vi "MultiPAS-UV-roll.vi"() -> ()   [LabVIEW 2011]
uses:
  sub/crd/fit/Analysis/analys_meth.ctl
  <vilib>/Analysis/4window.llb/windowTd.ctl
  sub/QMH/QMH Add Message to Queue (Single Element).vi
  sub/QMH/QMH Add Message to Queue (Array).vi
  sub/laserDiagnose_UV.vi
  <vilib>/Instr/_visa.llb/VISA Configure Serial Port (Instr).vi
  <vilib>/Utility/file.llb/Write To Spreadsheet File (string).vi
  sub/fftGetMags.vi
  sub/rollingAverage_III.vi
  sub/pdNormalize_III.vi
  <vilib>/measure/maspectr.llb/FFT Spectrum (Mag-Phase) for 1 Chan.vi
  sub/absCalcPlot_UV.vi
  sub/micUnbundle_III.vi
  <vilib>/measure/NI_MAPro.lvlib
  <vilib>/Analysis/NI_AALPro.lvlib
panel:
  out "x 2":dbl
  in  "x":dbl
  in  "y":dbl
  out "Chopper On":bool=TRUE caption="Overtemp"
  in  "Chopper":bool=TRUE
  in  "save spectrum":bool
  out "PAS Save":bool caption="Overtemp"
  in  "Data 2":i32[][](array[numeric])=[[-16374, -7248, 2543, 12030, 20279, 26487, 30037, 30583, 28073, 22744, 15131, 5976, -3818, -13288, -21504, -27663, -31155, -31636, -29064, -23686, -16036, -6862, 2936, 12388, 20571, 26684, 30122, 30546, 27911, 22483, 14793, 5595, -4207, -13644, -21795, -27855, -31232, -31591, -28898, -23423, -15695, -6476, 3323, 12743, 20858, 26873, 30194, 30492, 27744, 22213, 14447, 5207, -4597, -14002, -22082, -28044, -31304, -31540, -28731, -23149, -15348, -6093, 3713, 13101, 21145, 27063, 30265, 30442, 27576, 21943, 14103, 4822, -4984, -14354, -22365, -28230, -31373, -31485, -28556, -22876, -14998, -5702, 4104, 13452, 21428, 27245, 30335, 30388, 27400, 21669, 13754, 4435, -5375, -14705, -22643, -28407, -31436, -31426, -28378, -22598, -14648, -5314, 4497, 13803, 21706, 27423, 30394, 30325, 27221, 21390, 13402, 4045, -5763, -15056, -22921, -28586, -31496, -31361, -28198, -22319, -14297, -4924, 4879, 14151, 21982, 27597, 30451, 30257, 27038, 21107, 13050, 3658, -6149, -15402, -23193, -28754, -31546, -31290, -28010, -22033, -13944, -4536, 5266, 14498, 22252, 27767, 30500, 30184, 26849, 20821, 12696, 3267, -6535, -15748, -23462, -28924, -31596, -31216, -27821, -21748, -13587, -4147, 5653, 14838, 22519, 27930, 30549, 30110, 26658, 20535, 12337, 2878, -6919, -16089, -23727, -29087, -31641, -31137, -27627, -21457, -13229, -3753, 6038, 15181, 22786, 28093, 30591, 30031, 26461, 20243, 11979, 2485, -7303, -16428, -23991, -29244, -31678, -31053, -27426, -21159, -12867, -3360, 6424, 15524, 23043, 28252, 30633, 29946, 26262, 19946, 11617, 2096, -7686, -16764, -24246, -29398, -31712, -30964, -27224, -20862, -12503, -2971, 6803, 15859, 23301, 28401, 30661, 29852, 26058, 19648, 11254, 1703, -8069, -17099, -24500, -29547, -31741, -30870, -27018, -20562, -12138, -2575, 7188, 16192, 23556, 28549, 30689, 29756, 25848, 19348, 10891, 1312, -8448, -17430, -24753, -29691, -31765, -30773, -26806, -20259, -11775, -2186, 7566, 16521, 23801, 28690, 30709, 29656, 25634, 19038, 10523, 919, -8831, -17762, -24997, -29833, -31788, -30672, -26593, -19955, -11409, -1792, 7944, 16850, 24047, 28830, 30724, 29548, 25416, 18729, 10152, 523, -9212, -18092, -25245, -29969, -31805, -30566, -26375, -19647, -11041, -1403, 8319, 17173, 24287, 28963, 30734, 29436, 25192, 18418, 9781, 130, -9587, -18413, -25481, -30101, -31814, -30449, -26150, -19332, -10666, -1007, 8697, 17497, 24524, 29090, 30745, 29325, 24968, 18105, 9408, -263, -9962, -18735, -25718, -30228, -31820, -30334, -25921, -19016, -10296, -618, 9072, 17814, 24756, 29213, 30746, 29202, 24738, 17787, 9036, -657, -10338, -19058, -25951, -30350, -31818, -30214, -25690, -18699, -9922, -224, 9442, 18128, 24984, 29330, 30738, 29078, 24502, 17466, 8658, -1050, -10710, -19371, -26178, -30467, -31814, -30088, -25458, -18382, -9550, 167, 9812, 18440, 25206, 29443, 30732, 28947, 24264, 17143, 8281, -1445, -11083, -19685, -26404, -30581, -31807, -29959, -25221, -18059, -9175, 556, 10178, 18750, 25426, 29548, 30718, 28809, 24018, 16812, 7901, -1842, -11457, -19996, -26624, -30690, -31795, -29824, -24980, -17733, -8799, 950, 10549, 19058, 25643, 29655, 30700, 28673, 23773, 16484, 7523, -2235, -11824, -20304, -26840, -30793, -31772, -29682, -24731, -17402, -8415, 1341, 10916, 19363, 25856, 29755, 30677, 28528, 23522, 16151, 7141, -2626, -12191, -20607, -27051, -30891, -31746, -29536, -24481, -17070, -8035, 1733, 11280, 19664, 26064, 29851, 30648, 28381, 23272, 15818, 6762, -3019, -12555, -20906, -27258, -30984, -31717, -29391, -24226, -16736, -7655, 2128, 11641, 19962, 26270, 29940, 30615, 28229, 23013, 15483, 6376, -3409, -12914, -21204, -27459, -31071, -31684, -29236, -23967, -16398, -7271, 2515, 12005, 20258, 26468, 30024, 30577, 28072, 22753, 15143, 5990, -3802, -13276, -21497, -27660, -31157, -31643, -29076, -23707, -16058, -6886, 2908, 12363, 20550, 26666, 30107, 30536, 27914, 22489, 14805, 5607, -4192, -13633, -21787, -27849, -31230, -31597, -28911, -23438, -15716, -6501, 3298, 12719, 20839, 26858, 30182, 30488, 27744, 22223, 14459, 5225, -4579, -13988, -22071, -28040, -31304, -31549, -28743, -23167, -15368, -6113, 3693, 13076, 21126, 27047, 30255, 30438, 27576, 21950, 14113, 4837, -4971, -14340, -22354, -28224, -31375, -31494, -28570, -22895, -15022, -5725, 4080, 13430, 21408, 27230, 30324, 30384, 27402, 21676, 13766, 4449, -5360, -14694, -22636, -28409, -31440, -31436, -28397, -22617, -14674, -5338, 4467, 13781, 21686, 27408, 30385, 30320, 27224, 21398, 13418, 4062, -5748, -15044, -22913, -28584, -31498, -31368, -28212, -22339, -14321, -4948, 4856, 14131, 21963, 27583, 30440, 30254, 27042, 21118, 13062, 3669, -6137, -15390, -23183, -28751, -31551, -31297, -28024, -22049, -13962, -4556, 5245, 14476, 22235, 27754, 30497, 30186, 26857, 20834, 12710, 3283, -6519, -15733, -23453, -28921, -31600, -31226, -27837, -21765, -13610, -4168, 5628, 14820, 22502, 27918, 30540, 30109, 26664, 20544, 12354, 2891, -6906, -16074, -23719, -29085, -31646, -31148, -27642, -21475, -13251, -3777, 6014, 15160, 22765, 28078, 30583, 30027, 26468, 20251, 11994, 2501, -7292, -16415, -23980, -29242, -31682, -31064, -27443, -21181, -12892, -3386, 6397, 15501, 23026, 28238, 30624, 29944, 26269, 19959, 11633, 2110, -7673, -16753, -24239, -29395, -31719, -30974, -27239, -20882, -12528, -2993, 6782, 15835, 23285, 28390, 30651, 29852, 26063, 19660, 11271, 1720, -8053, -17087, -24493, -29546, -31746, -30880, -27031, -20583, -12163, -2599, 7166, 16173, 23538, 28538, 30684, 29758, 25853, 19356, 10906, 1327, -8433, -17416, -24743, -29688, -31769, -30782, -26821, -20280, -11797, -2208, 7543, 16501, 23786, 28680, 30704, 29656, 25642, 19053, 10540, 936, -8814, -17747, -24989, -29827, -31787, -30678, -26606, -19973, -11430, -1817, 7923, 16829, 24031, 28819, 30721, 29552, 25424, 18746, 10174, 543, -9191, -18072, -25231, -29962, -31802, -30567, -26384, -19660, -11057, -1422, 8302, 17159, 24274, 28952, 30738, 29443, 25205, 18435, 9801, 150, -9568, -18401, -25472, -30095, -31811, -30457, -26163, -19349, -10687, -1031, 8679, 17481, 24511, 29082, 30742, 29327, 24979, 18121, 9431, -241, -9943, -18717, -25707, -30221, -31815, -30337, -25930, -19029, -10312, -631, 9058, 17802, 24745, 29207, 30746, 29209, 24750, 17805, 9057, -634, -10316, -19037, -25937, -30340, -31814, -30217, -25700, -18713, -9939, -240, 9429, 18117, 24976, 29328, 30740, 29088, 24519, 17486, 8682, -1027, -10688, -19352, -26164, -30458, -31810, -30091, -25465, -18390, -9561, 154, 9800, 18433, 25201, 29442, 30735, 28959, 24282, 17165, 8308, -1420, -11063, -19665, -26386, -30570, -31801, -29961, -25227, -18068, -9185, 547, 10171, 18745, 25424, 29552, 30726, 28825, 24038, 16835, 7925, -1815, -11429, -19974, -26608, -30681, -31789, -29826, -24984, -17741, -8807, 938, 10536, 19047, 25636, 29657, 30708, 28685, 23794, 16510, 7550, -2205, -11798, -20280, -26821, -30782, -31766, -29684, -24737, -17411, -8429, 1331, 10906, 19356, 25851, 29758, 30684, 28544, 23546, 16178, 7169, -2598, -12162, -20582, -27035, -30879, -31744, -29540, -24485, -17080, -8048, 1721, 11267, 19655, 26061, 29852, 30654, 28395, 23291, 15843, 6786, -2993, -12527, -20884, -27240, -30974, -31713, -29390, -24230, -16744, -7662, 2115, 11635, 19957, 26268, 29945, 30624, 28246, 23035, 15509, 6406, -3382, -12889, -21180, -27444, -31061, -31677, -29236, -23975, -16408, -7284], [-19329, -1252, 17344, 29341, 30145, 19451, 1353, -17227, -29174, -29920, -19175, -1056, 17506, 29408, 30095, 19300, 1159, -17387, -29238, -29860, -19019, -860, 17671, 29475, 30037, 19143, 960, -17553, -29307, -29809, -18866, -664, 17832, 29545, 29987, 18991, 771, -17707, -29365, -29749, -18707, -466, 17992, 29605, 29926, 18832, 570, -17873, -29434, -29694, -18556, -272, 18151, 29670, 29869, 18676, 375, -18031, -29495, -29633, -18395, -75, 18310, 29729, 29809, 18516, 175, -18194, -29561, -29579, -18238, 120, 18469, 29792, 29750, 18362, -17, -18347, -29617, -29515, -18076, 316, 18629, 29848, 29682, 18197, -218, -18510, -29679, -29456, -17921, 513, 18787, 29910, 29626, 18042, -408, -18664, -29734, -29388, -17757, 709, 18941, 29965, 29560, 17875, -609, -18823, -29791, -29326, -17600, 904, 19095, 30023, 29495, 17717, -802, -18975, -29845, -29260, -17434, 1099, 19251, 30075, 29425, 17551, -1001, -19131, -29901, -29194, -17277, 1296, 19408, 30130, 29359, 17393, -1193, -19284, -29953, -29124, -17112, 1491, 19560, 30184, 29290, 17225, -1392, -19440, -30008, -29056, -16949, 1686, 19713, 30237, 29226, 17069, -1581, -19587, -30054, -28982, -16781, 1883, 19866, 30287, 29151, 16898, -1781, -19742, -30107, -28913, -16616, 2079, 20018, 30337, 29082, 16737, -1973, -19888, -30152, -28838, -16449, 2275, 20167, 30383, 29006, 16564, -2174, -20041, -30200, -28765, -16282, 2471, 20321, 30430, 28934, 16403, -2364, -20187, -30243, -28688, -16113, 2669, 20465, 30470, 28853, 16230, -2568, -20341, -30294, -28618, -15953, 2860, 20615, 30519, 28783, 16070, -2755, -20486, -30335, -28537, -15779, 3057, 20760, 30560, 28700, 15892, -2956, -20637, -30378, -28461, -15613, 3252, 20909, 30605, 28628, 15730, -3145, -20777, -30418, -28377, -15440, 3446, 21054, 30645, 28543, 15557, -3345, -20927, -30460, -28299, -15271, 3643, 21199, 30686, 28465, 15391, -3534, -21066, -30495, -28215, -15100, 3839, 21345, 30722, 28380, 15214, -3734, -21213, -30534, -28134, -14928, 4032, 21487, 30760, 28300, 15044, -3926, -21355, -30570, -28052, -14757, 4225, 21627, 30792, 28209, 14870, -4123, -21501, -30607, -27968, -14586, 4419, 21768, 30832, 28129, 14702, -4314, -21637, -30639, -27880, -14413, 4612, 21907, 30859, 28040, 14521, -4515, -21780, -30675, -27796, -14241, 4804, 22048, 30895, 27953, 14352, -4702, -21919, -30705, -27707, -14064, 4999, 22187, 30922, 27859, 14172, -4900, -22060, -30739, -27620, -13892, 5193, 22326, 30954, 27773, 14003, -5090, -22194, -30765, -27524, -13712, 5386, 22462, 30981, 27679, 13823, -5285, -22333, -30794, -27436, -13538, 5580, 22600, 31013, 27591, 13650, -5476, -22466, -30820, -27343, -13363, 5770, 22732, 31033, 27491, 13468, -5673, -22605, -30848, -27251, -13187, 5964, 22870, 31060, 27401, 13292, -5863, -22736, -30870, -27155, -13010, 6156, 23000, 31079, 27299, 13111, -6058, -22873, -30895, -27060, -12833, 6347, 23134, 31104, 27208, 12936, -6248, -23004, -30918, -26965, -12652, 6536, 23260, 31120, 27106, 12753, -6444, -23136, -30939, -26865, -12472, 6729, 23395, 31148, 27011, 12578, -6634, -23266, -30959, -26766, -12296, 6919, 23523, 31161, 26907, 12392, -6830, -23402, -30982, -26665, -12115, 7109, 23652, 31180, 26809, 12213, -7016, -23524, -30992, -26564, -11932, 7301, 23777, 31195, 26704, 12032, -7210, -23655, -31011, -26464, -11755, 7492, 23907, 31211, 26605, 11855, -7395, -23778, -31024, -26358, -11573, 7680, 24031, 31218, 26494, 11665, -7592, -23908, -31039, -26258, -11392, 7871, 24158, 31237, 26394, 11491, -7775, -24031, -31050, -26153, -11210, 8063, 24281, 31247, 26285, 11302, -7972, -24159, -31062, -26046, -11027, 8250, 24407, 31258, 26180, 11124, -8157, -24276, -31067, -25937, -10841, 8438, 24526, 31265, 26071, 10936, -8347, -24401, -31078, -25829, -10659, 8630, 24649, 31275, 25965, 10755, -8533, -24522, -31087, -25721, -10474, 8816, 24770, 31280, 25853, 10566, -8726, -24641, -31091, -25608, -10290, 9003, 24891, 31287, 25746, 10386, -8910, -24756, -31095, -25498, -10105, 9192, 25008, 31287, 25627, 10196, -9102, -24881, -31101, -25386, -9919, 9381, 25127, 31296, 25521, 10019, -9284, -24994, -31099, -25268, -9732, 9570, 25243, 31293, 25403, 9826, -9476, -25113, -31105, -25157, -9544, 9756, 25359, 31298, 25291, 9645, -9655, -25225, -31099, -25040, -9359, 9942, 25473, 31291, 25167, 9453, -9847, -25341, -31102, -24926, -9173, 10124, 25586, 31294, 25057, 9269, -10029, -25450, -31095, -24809, -8986, 10310, 25696, 31284, 24931, 9078, -10218, -25564, -31094, -24688, -8798, 10497, 25812, 31287, 24819, 8896, -10399, -25673, -31085, -24567, -8608, 10682, 25922, 31278, 24698, 8703, -10587, -25785, -31080, -24448, -8422, 10866, 26033, 31274, 24582, 8522, -10765, -25890, -31067, -24321, -8230, 11050, 26140, 31263, 24455, 8325, -10952, -26001, -31064, -24201, -8040, 11234, 26248, 31255, 24338, 8142, -11132, -26106, -31054, -24079, -7852, 11417, 26353, 31243, 24207, 7948, -11316, -26217, -31041, -23952, -7662, 11601, 26464, 31236, 24089, 7763, -11494, -26315, -31025, -23829, -7471, 11782, 26562, 31217, 23957, 7567, -11682, -26422, -31014, -23702, -7282, 11962, 26667, 31205, 23834, 7383, -11859, -26521, -30998, -23575, -7092, 12144, 26770, 31187, 23704, 7186, -12043, -26626, -30981, -23444, -6900, 12328, 26875, 31176, 23582, 7003, -12218, -26724, -30962, -23316, -6709, 12505, 26971, 31154, 23446, 6805, -12401, -26825, -30946, -23189, -6517, 12687, 27073, 31139, 23322, 6620, -12576, -26919, -30922, -23054, -6323, 12867, 27170, 31114, 23185, 6422, -12760, -27022, -30904, -22923, -6132, 13047, 27272, 31096, 23060, 6237, -12934, -27114, -30879, -22790, -5940, 13222, 27362, 31068, 22921, 6041, -13116, -27212, -30855, -22657, -5748, 13401, 27461, 31048, 22790, 5853, -13289, -27302, -30828, -22522, -5555, 13577, 27549, 31019, 22652, 5652, -13472, -27398, -30806, -22388, -5362, 13753, 27645, 30995, 22521, 5463, -13642, -27487, -30776, -22248, -5169, 13928, 27733, 30963, 22376, 5266, -13823, -27584, -30750, -22113, -4975, 14106, 27828, 30937, 22246, 5082, -13992, -27669, -30717, -21974, -4782, 14280, 27914, 30902, 22101, 4880, -14174, -27760, -30689, -21837, -4588, 14454, 28006, 30875, 21965, 4692, -14340, -27843, -30653, -21693, -4391, 14631, 28092, 30840, 21822, 4494, -14519, -27934, -30620, -21552, -4198, 14805, 28179, 30808, 21688, 4308, -14687, -28015, -30582, -21410, -4004, 14975, 28262, 30770, 21540, 4106, -14861, -28103, -30548, -21268, -3808, 15149, 28349, 30739, 21402, 3916, -15032, -28183, -30512, -21124, -3614, 15319, 28430, 30697, 21255, 3715, -15205, -28267, -30475, -20982, -3421, 15490, 28513, 30664, 21116, 3524, -15376, -28348, -30435, -20837, -3225, 15660, 28592, 30617, 20962, 3327, -15550, -28432, -30397, -20695, -3032, 15829, 28673, 30581, 20820, 3134, -15711, -28506, -30353, -20546, -2837, 15994, 28746, 30530, 20669, 2933, -15887, -28585, -30311, -20400, -2641, 16167, 28828, 30496, 20528, 2745, -16052, -28660, -30264, -20248, -2445, 16335, 28901, 30445, 20376, 2544, -16221, -28737, -30219, -20102, -2250, 16505, 28983, 30406, 20231, 2357, -16381, -28808, -30171, -19950, -2053, 16670, 29053, 30355, 20075, 2154, -16552, -28883, -30127, -19803, -1859, 16835, 29128, 30308, 19930, 1965, -16714, -28952, -30073, -19650, -1663, 17001, 29192, 30255, 19772, 1764, -16881, -29028, -30026, -19496, -1467, 17165, 29268, 30208, 19626, 1572, -17043, -29095, -29977, -19346]]
  out "Filtering":bool caption="Time has Elapsed"
  in  "Switch Filter":bool
  in  "Auto Filter":bool
  out "Elapsed Time (min)":dbl caption="Elapsed Time (s)" format="%#.1g"
  in  "Filter Length (min)":dbl=6.0 caption="Time Target (s)"
  in  "Sample Length (min)":dbl=24.0 caption="Time Target (s)" format="%#.1f"
  out "Time has Elapsed":bool
  in  "Time Target (s)":dbl=1.0
  in  "All Emit":bool
  in  "Alignment Mode":bool
  in  "445 Emission":bool
  in  "445 Power (mW)":dbl(slide)=75.0 min=0.0 max=75.0 step=1.0 scale=0.0..75.0
  in  "375 Emission":bool
  in  "375 Power (mW)":dbl(slide)=100.0 min=0.0 max=50.0 step=1.0 scale=0.0..50.0
  in  "320 Emission":bool=TRUE
  out "Overtemp":bool
  in  "Tab Control":T1(tab)=enum."Oscilloscope"
  out "Laser Currents":T2(graph)
  in  "Chopper Port":refnum<visa-resource-name>="COM6"
  out "sweeps":path caption="Microphone File Path"
  in  "save interval (ms)":u32=1000
  out "Error Console":T3
  out "pas":path caption="Microphone File Path"
  out "Laser Temperatures":T2(graph)
  in  "pd id":u32=2
  in  "mic id":u32
  in  "mic cal, scu":dbl=5.41531278804282e-05 format="%#_3e"
  in  "mic cal, scu":dbl=5.59307241877627e-05 format="%#_3e"
  in  "320 Port":refnum<visa-resource-name>="COM5"
  in  "375 Port":refnum<visa-resource-name>="COM14"
  in  "445 Port":refnum<visa-resource-name>="COM13"
  in  "Teensy Port":refnum<visa-resource-name>="COM12"
  in  "Save Data":bool
  in  "405 PD Cal 3":dbl=0.039
  in  "532 PD Cal 3":dbl=0.0348
  in  "660 PD Cal 3":dbl=0.2015
  out "Laser Powers":T2(graph)
  in  "tau Rolling Avg":i32=8
  out "error out":errorcluster
  in  "Channel B Settings":T4={"Enabled"=TRUE, "Coupling"=1, "Range"=8, "Analogue Offset"=0.0} {"Range" items=["20 mV"=1, "50 mV"=2, "100 mV"=3, "200 mV"=4, "500 mV"=5, "1 V"=6, "2 V"=7, "5 V"=8, "10 V"=9, "20 V"=10]; "Coupling" items=["AC", "DC"]}
  in  "Rapid Block Acquisition Settings":T5={"preTriggerSamples"=0, "postTriggerSamples"=90000, "timebase"=1, "Down-Sample Mode"=4, "Down Sample Ratio"=10, "Oversample"=1, "Number of Captures"=100} {"Down Sample Ratio" min=1 step=1; "Down-Sample Mode" items=["None"=0, "Aggregate"=1, "Decimate"=2, "Average"=4]}
  in  "crd delay":u32=1000
  in  "Trigger Settings":T6={"Trigger Enabled"=TRUE, "Trigger Source"=enum."Channel B", "Trigger Threshold (Volts)"=1.0, "Trigger Direction"=3, "Trigger Delay (samples)"=0, "Auto Trigger Time (ms)"=1000} {"Trigger Direction" items=["Rising"=2, "Falling"=3]}
  in  "Channel A Settings":T4={"Enabled"=TRUE, "Coupling"=0, "Range"=3, "Analogue Offset"=0.0} {"Range" items=["20 mV"=1, "50 mV"=2, "100 mV"=3, "200 mV"=4, "500 mV"=5, "1 V"=6, "2 V"=7, "5 V"=8, "10 V"=9, "20 V"=10]; "Coupling" items=["AC", "DC"]}
  in  "factor":sgl=10.0
  in  "sweep":bool
  out "freqscan":cluster{i32[], "Best Gaussian Fit":dbl[]}[](graph) caption="Frequency Sweep"
  out "sweep progress":dbl(slide) scale=0.0..1.0
  in  "Autosweep?":bool=TRUE
  in  "set freqs":bool
  out "Calculated Resonance (Hz)":dbl=1370.0
  in  "Data Start Frequency (Hz)":i32=1355
  in  "Data End Frequency (Hz)":i32=1405
  in  "320 F (Hz)":i32=1368
  in  "375 F (Hz)":i32=1372
  in  "445 F (Hz)":i32=1370
  in  "Chart Rolling Average":i32=16
  out "pdwave":waveform(i32)(graph) caption="Photodiode Waveform"
  out "pd ts":cluster{dbl, dbl, dbl}(graph)
  out "pdfft":cluster{"f0":dbl, "df":dbl, "magnitude":dbl[]}(graph) caption="Photodiode FFT"
  in  "rollavg":i32=16 caption="Dispaly Averaging (Transfers to Absorption Data!)"
  out "mic ts":T7(graph)
  out "micfft":cluster{"f0":dbl, "df":dbl, "magnitude":dbl[]}(graph) caption="Photodiode FFT"
  out "micwave":waveform(i32)(graph) caption="Photodiode Waveform"
  in  "tau0":dbl
  in  "getbkg":bool
  out "AAE":dbl(graph)
  in  "Bkg Values (mV)":cluster{dbl, dbl, dbl}
  out "Absorption Spectrum":cluster{dbl[], "Best Power Fit":dbl[]}[](graph)
  in  "cellcal":dbl=95000.0 caption="Cell Calibration Coefficient (mV/mW)"
  out "abs/ext":cluster{dbl, dbl, dbl, "b_ext (1/Mm)":dbl}(graph)
  out "tau":dbl(graph)
  out "decay":cluster{i32, dbl, "Data (mV)":dbl[]}[](graph)
  out "Status":string
  in  "Exit":bool
  in  "State Variables":cluster{"CurrentFile":path}
  # "MultiPAS-UV | AeroSmith Labs (2017)"
  # "Laser Control"
  # "Filter Control"
  # "Communications"
  # "Sound Card Parameters"
  # "Data File Options"
  # "File paths are populated automatically at <...\\My Documents\\MultiPAS Data\\>.  To save in another location, turn on \"Save Data\" and follow the prompts to choose an alternate working directory."
  # "Photodiode Calibration"
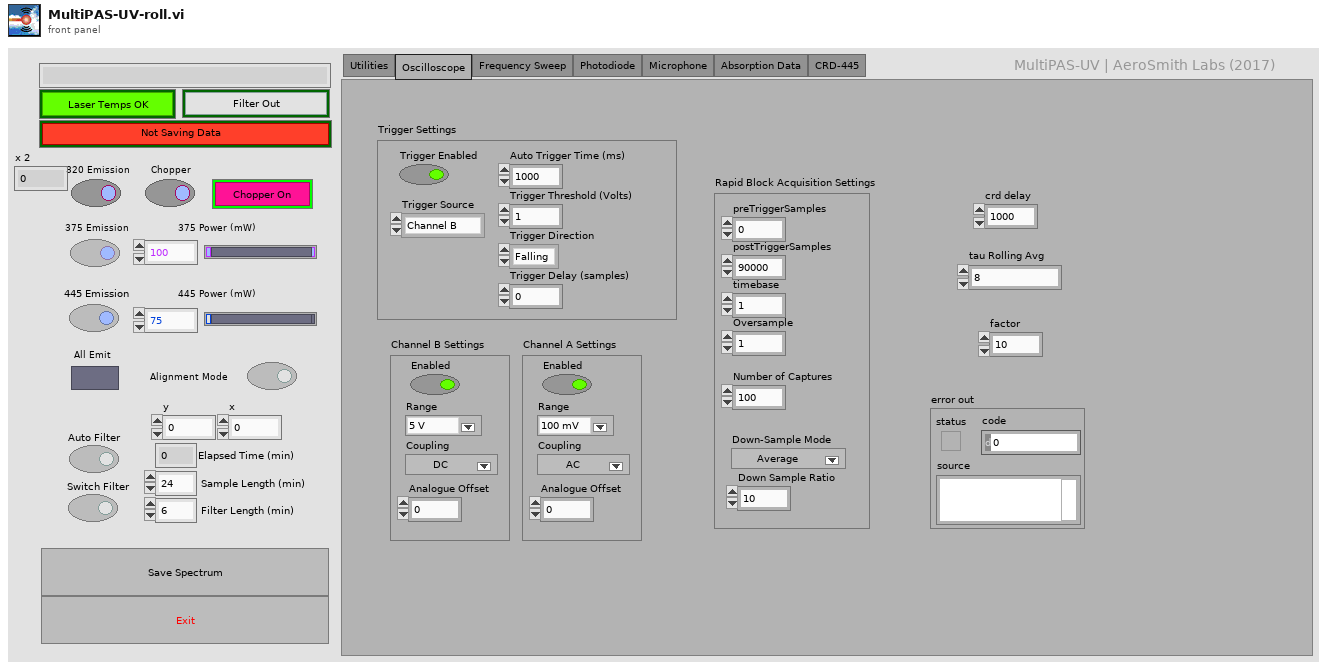
[diagram p1: front panel]
types:
  T1 = enum32{"Utilities", "Oscilloscope", "Frequency Sweep", "Photodiode", "Microphone", "Absorption Data", "CRD-445"}
  T2 = cluster{"Temp (C)":dbl, "Temp (C)":dbl, "Temp (C)":dbl}
  T3 = cluster{"status":bool, "code":i32, "Message":string}
  T4 = cluster{"Enabled":bool, "Coupling":i16, "Range":u16, "Analogue Offset":sgl}
  T5 = cluster{"preTriggerSamples":u32, "postTriggerSamples":u32, "timebase":u32, "Down-Sample Mode":i32, "Down Sample Ratio":u32, "Oversample":i16, "Number of Captures":u32}
  T6 = cluster{"Trigger Enabled":bool, "Trigger Source":enum16{"Channel A", "Channel B", "Channel C", "Channel D", "Ext."}, "Trigger Threshold (Volts)":dbl, "Trigger Direction":u16, "Trigger Delay (samples)":u32, "Auto Trigger Time (ms)":i16}
  T7 = cluster{"422 Mean":dbl, "532 Mean":dbl, "785 Mean":dbl}
  T8 = cluster{"# buffers":i32, "Buffer size":i32, "unit (ms)":enum16{"time (ms)", "Samples"}}
  T9 = typedef "SoundHandle.ctl" = cluster{"DeviceID":u16, "Samples/buf":u32, "Sampl rate":u32, "Bits/sample":u16, "Channels":u8, "Opened":bool}
  T10 = cluster{"Output Power at Laser Head":dbl, "Output Power at Laser Head":dbl, "Output Power at Laser Head":dbl}
  T11 = cluster{"Current (mA)":dbl, "Current (mA)":dbl, "Current (mA)":dbl}
  T12 = cluster{"405 Mean":dbl, "532 Mean":dbl, "660 Mean":dbl}
  T13 = typedef "NI_AALPro.lvlib/windowTd.ctl" = u32
  T14 = cluster{"785 New Array":dbl[], "785 Mean":dbl, "785 SD":dbl}
  T15 = cluster{"532 New Array":dbl[], "532 Mean":dbl, "532 SD":dbl}
  T16 = cluster{"422 New Array":dbl[], "422 Mean":dbl, "422 SD":dbl}
  T17 = typedef "analys_meth.ctl" = enum16{"DFT-1", "DFT-5", "LRS"}
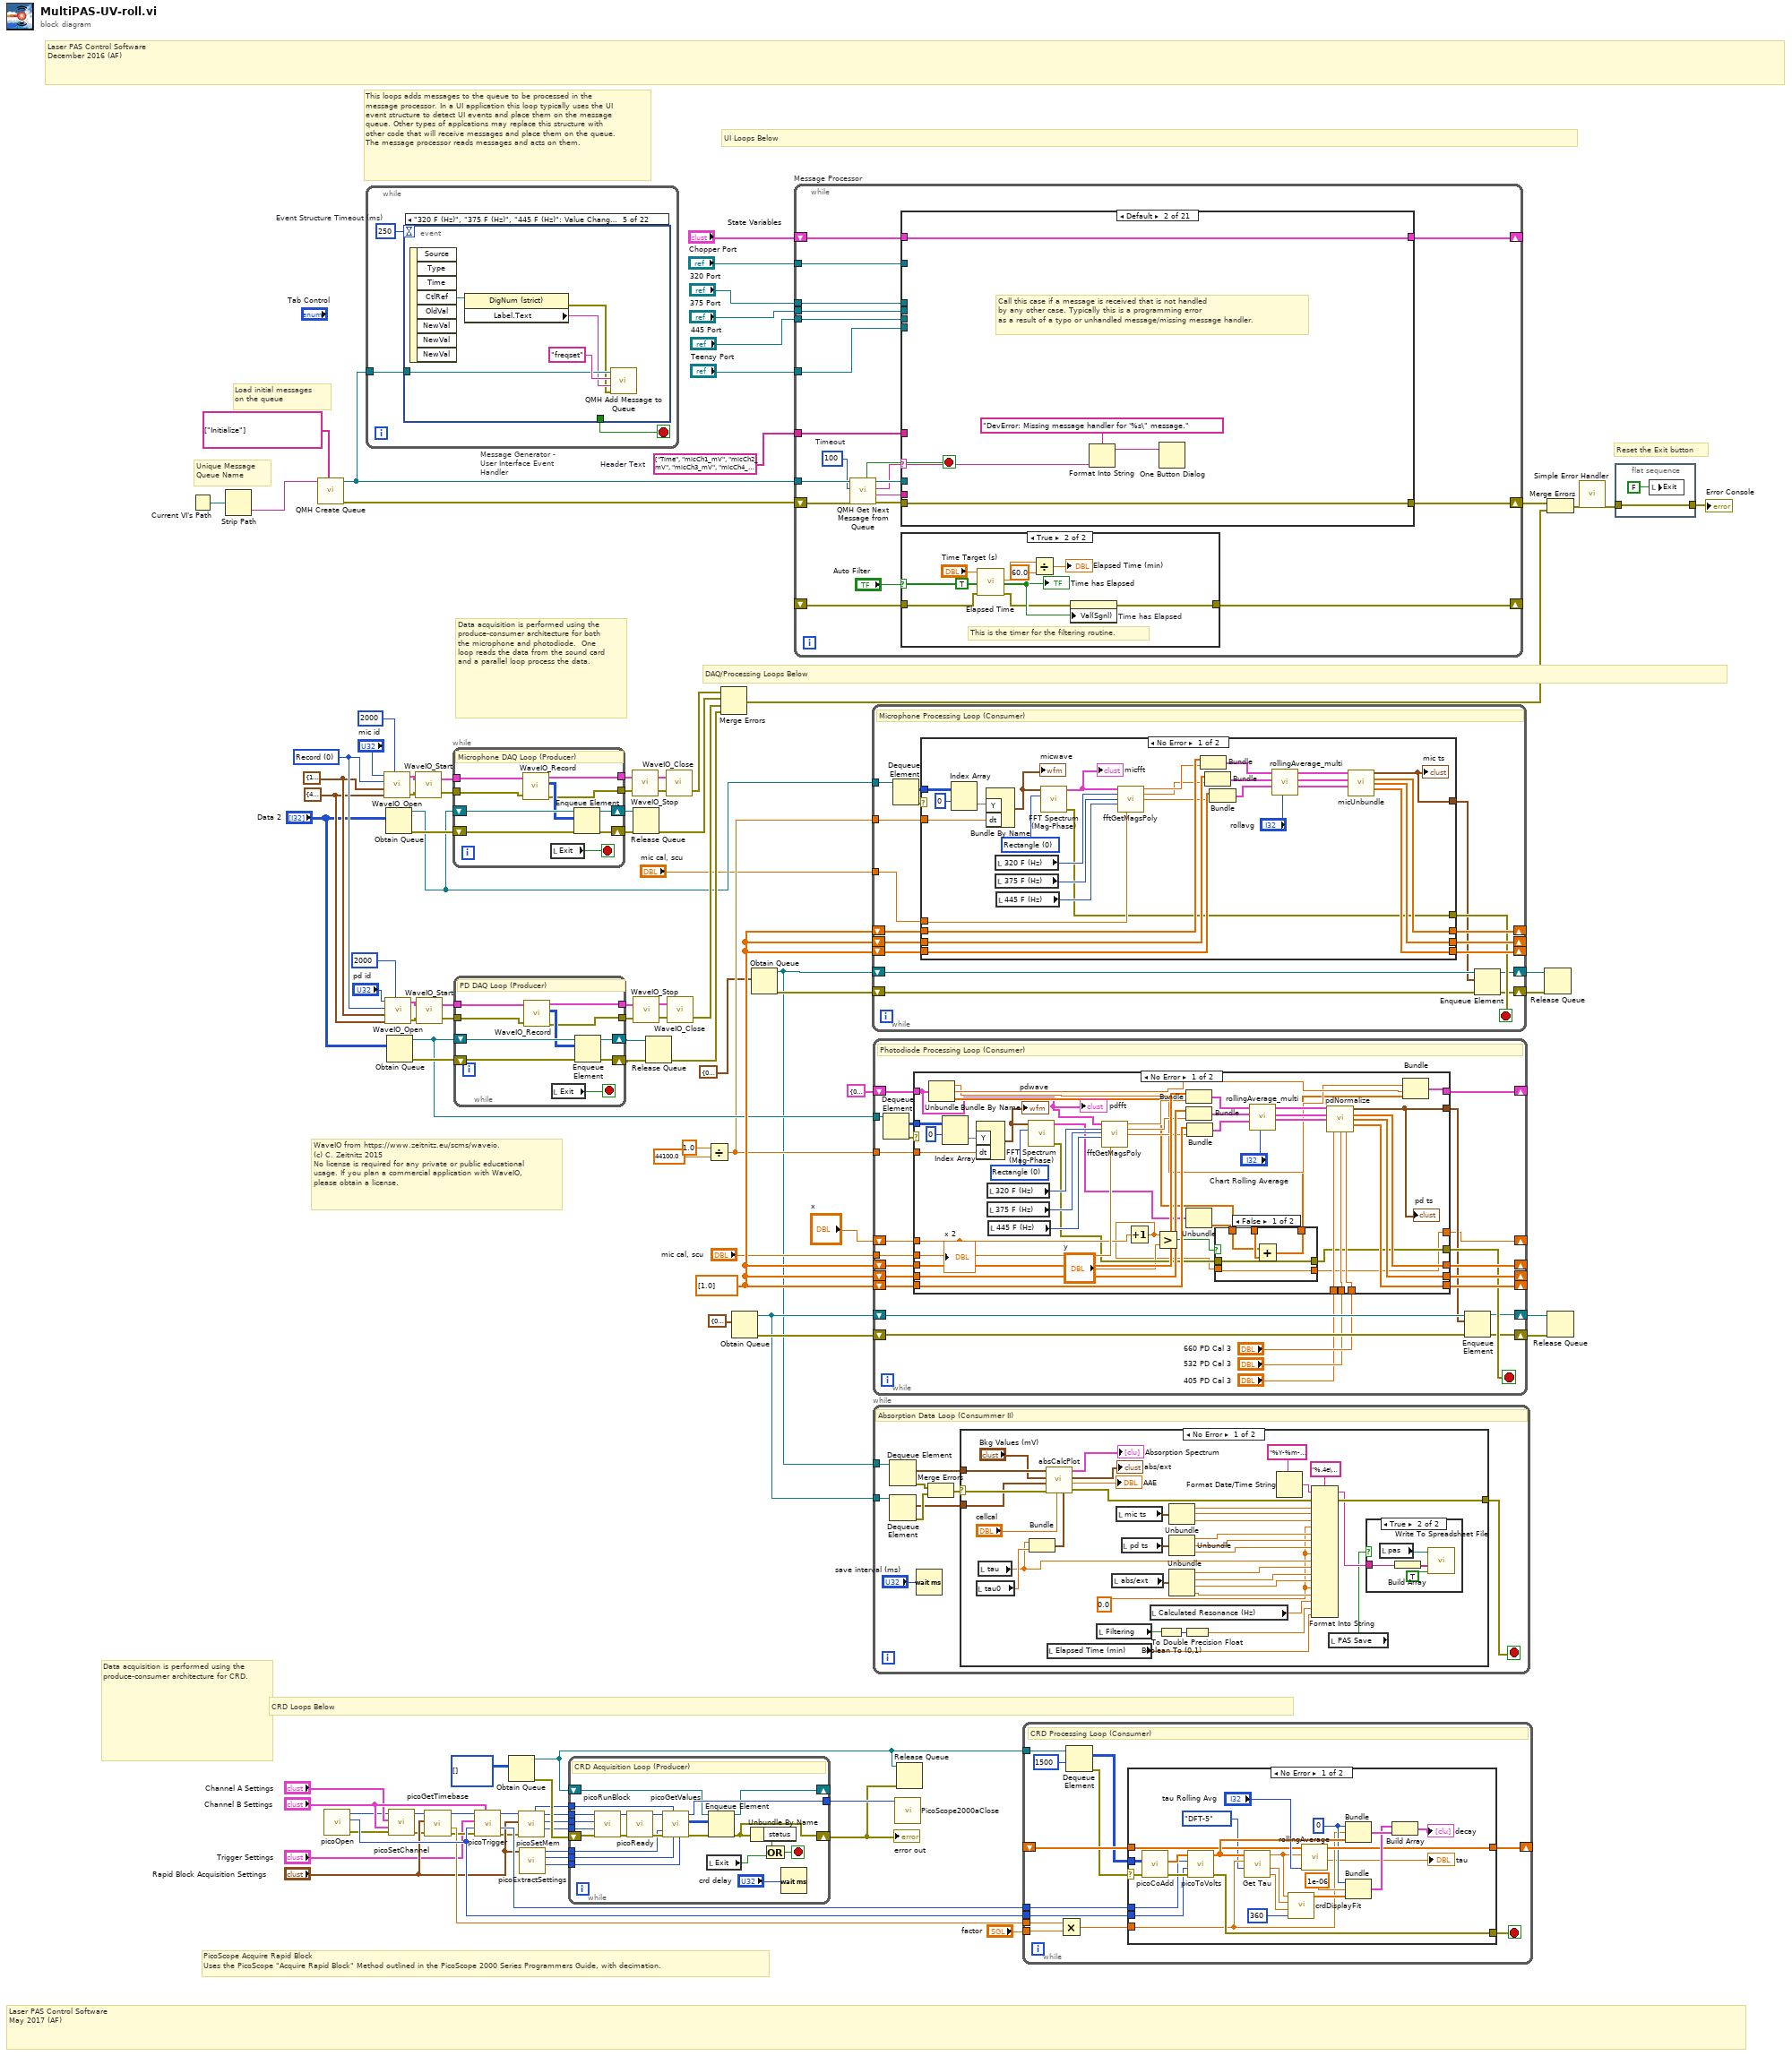
[diagram p0: block diagram]
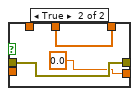
[diagram p5: hidden frame]
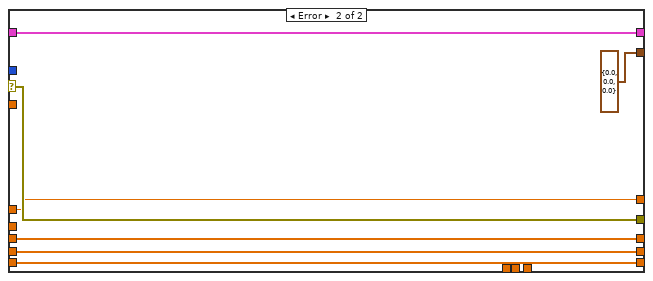
[diagram p6: hidden frame]
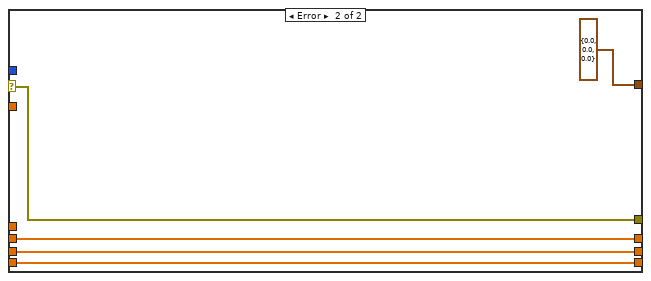
[diagram p7: hidden frame]
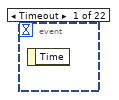
[diagram p8: hidden frame]
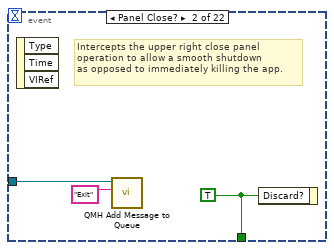
[diagram p9: hidden frame]
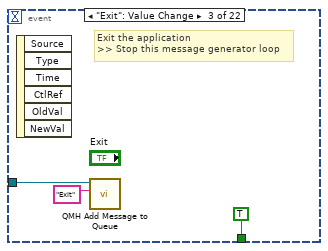
[diagram p10: hidden frame]
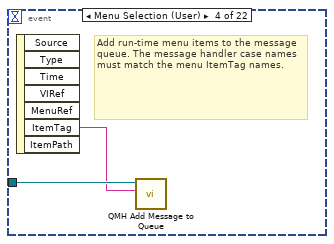
[diagram p11: hidden frame]
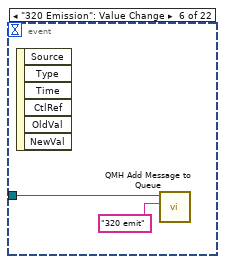
[diagram p12: hidden frame]
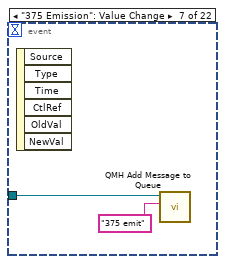
[diagram p13: hidden frame]
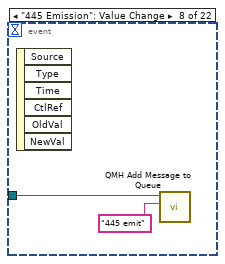
[diagram p14: hidden frame]
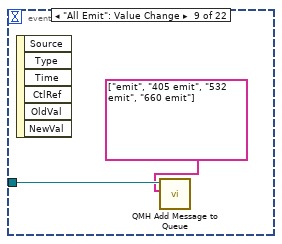
[diagram p15: hidden frame]
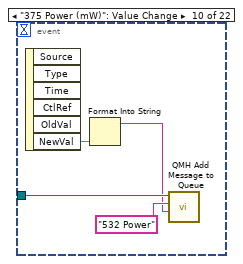
[diagram p16: hidden frame]
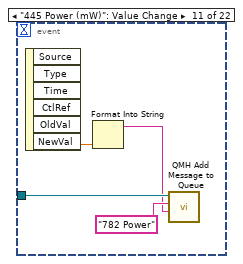
[diagram p17: hidden frame]
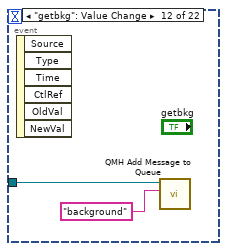
[diagram p18: hidden frame]
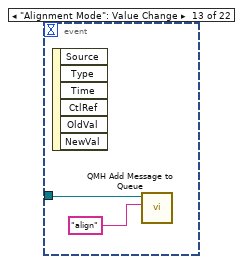
[diagram p19: hidden frame]
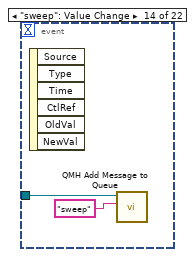
[diagram p20: hidden frame]
diagram:
  w32 = string[] ["Time", "micCh1_mV", "micCh2_mV", "micCh3_mV", "micCh4_mV", "pdCh1_mV", "pdCh2_mV", "pdCh3_mV", "pdCh4_mV", "tau_sec", "babsCh1_Mm", "babsCh2_Mm", "babsCh3_Mm", "babsCh4_Mm", "bext_Mm", "fres_Hz", "filter_state", "elapsedTime_min"]  # Header Text
  w52 = T8 {"# buffers"=10, "Buffer size"=44100, "unit (ms)"=enum."Samples"} ("Buffer")
  w51 = cluster{"Rate":i32, "Bits":i32, "Channels":i32} {"Rate"=44100, "Bits"=24, "Channels"=2} ("Format")
  w53 = u16 0 items=["Record", "Play", "Loopback", "ASIO input", "ASIO output"] ("Direction (Record)")
  w83 = dbl[] [1.0] ("X")
  # "PicoScope Acquire Rapid Block\nUses the PicoScope \"Acquire Rapid Block\" Method outlined in the PicoScope 2000 Series Programmers Guide, with decimation."
  # "Data acquisition is performed using the produce-consumer architecture for CRD."
  # "CRD Loops Below"
  # "Laser PAS Control Software\nMay 2017 (AF)"
  # "Laser PAS Control Software\nDecember 2016 (AF)"
  # "Data acquisition is performed using the produce-consumer architecture for both the microphone and photodiode.  One loop reads the data from the sound card and a parallel loop process the data."
  # "WaveIO from https://www.zeitnitz.eu/scms/waveio.\n(c) C. Zeitnitz 2015\nNo license is required for any private or public educational usage. If you plan a commercial application with WaveIO, please obtain a license."
  # "This loops adds messages to the queue to be processed in the message processor. In a UI application this loop typically uses the UI event structure to detect UI events and place them on the message queue. Other types of applcations may replace this structure with other code that will receive messages and place them on the queue.  The message processor reads messages and acts on them."
  # "Reset the Exit button"
  # "Unique Message\nQueue Name"
  # "Load initial messages\non the queue"
  # "DAQ/Processing Loops Below"
  # "UI Loops Below"
  n1 = Current VI's Path() -> (path=w98:path)
  n2 = Strip Path(path=w98) -> (name=w99:string)  [unwired: 1 out]
  n3 = call "QMH Create Queue.vi"("Initial Messages"=string[] ["Initialize"], "Message queue name (unnamed)"=w99) -> ("error out"=w95:errorcluster, "queue out"=w80:refnum<queue>)  [unwired: 8 in]
  n4 = call "picoOpen.vi"() -> ("error out"=w7:errorcluster, "maxADC"=w26:i16, "Handle Out"=w6:i16)  [unwired: 8 in, 1 out]
  n5 = while "Message Generator - User Interface Event Handler" {
    tunnel: w80 -> [w100]
    stop <- w101 stop-if-true
    w102 = 250  # Event Structure Timeout (ms)
    n6 = event shown="[4] \"320 F (Hz)\", \"375 F (Hz)\", \"445 F (Hz)\": Value Change" {
      selector: _ -> [_ _ _ _ _ _ _ _ _ _ _ _ _ _ _ _ _ _ _ _ _ _]
      dyn-events: _ -> [_ _ _ _ _ _ _ _ _ _ _ _ _ _ _ _ _ _ _ _ _ _]
      timeout: w102 -> [_ _ _ _ _ _ _ _ _ _ _ _ _ _ _ _ _ _ _ _ _ _]
      tunnel: [_ w105 TRUE ("Discard?") _ _ _ _ _ _ _ _ _ _ _ _ _ _ _ _ _ _ _] -> w101
      tunnel: w100 -> [_ w104 w107 w110 w114 w116 w118 w120 w123 w126 w130 w132 w134 w137 w141 w146 w151 w155 w160 w162 w164 w166]
      event Timeout {
        n7 = event-data() -> ()  [unwired: 1 in, 1 out]
      }
      event Panel Close? {
        w105 = TRUE ("Discard?")
        # "Intercepts the upper right close panel\noperation to allow a smooth shutdown\nas opposed to immediately killing the app."
        n8 = event-data() -> ()  [unwired: 1 in, 3 out]
        n9 = call-poly "QMH Add Message to Queue.vi"("Message"="Exit", "queue in"=w104) -> ()  [unwired: 8 in, 2 out]
        n10 = event-data("Discard?"=w105) -> ()  [unwired: 1 in, 1 out]
      }
      event "Exit": Value Change {
        # "Exit the application\n>> Stop this message generator loop"
        n11 = event-data() -> ()  [unwired: 1 in, 6 out]
        n12 = call-poly "QMH Add Message to Queue.vi"("Message"="Exit", "queue in"=w107) -> ()  [unwired: 8 in, 2 out]
      }
      event Menu Selection (User) {
        # "Add run-time menu items to the message\nqueue. The message handler case names must match the menu ItemTag names."
        n13 = event-data() -> ("ItemTag"=w109:string)  [unwired: 1 in, 6 out]
        n14 = call-poly "QMH Add Message to Queue.vi"("Message"=w109, "queue in"=w110) -> ()  [unwired: 8 in, 2 out]
      }
      event "320 F (Hz)", "375 F (Hz)", "445 F (Hz)": Value Change {
        n15 = event-data() -> ("CtlRef"=w113:refnum<vi>)  [unwired: 1 in, 7 out]
        n16 = property class="DigNum (strict)"(reference=w113) -> (error out=w111:errorcluster, "Label.Text"=w112:string)  [unwired: 1 in, 1 out]
        n17 = call-poly "QMH Add Message to Queue.vi"("error in (no error)"=w111, "Parameter"=w112, "Message"="freqset", "queue in"=w114) -> ()  [unwired: 6 in, 2 out]
      }
      event "320 Emission": Value Change {
        n18 = event-data() -> ()  [unwired: 1 in, 6 out]
        n19 = call-poly "QMH Add Message to Queue.vi"("Message"="320 emit", "queue in"=w116) -> ()  [unwired: 8 in, 2 out]
      }
      event "375 Emission": Value Change {
        n20 = event-data() -> ()  [unwired: 1 in, 6 out]
        n21 = call-poly "QMH Add Message to Queue.vi"("Message"="375 emit", "queue in"=w118) -> ()  [unwired: 8 in, 2 out]
      }
      event "445 Emission": Value Change {
        n22 = event-data() -> ()  [unwired: 1 in, 6 out]
        n23 = call-poly "QMH Add Message to Queue.vi"("Message"="445 emit", "queue in"=w120) -> ()  [unwired: 8 in, 2 out]
      }
      event "All Emit": Value Change {
        n24 = event-data() -> ()  [unwired: 1 in, 6 out]
        n25 = call-poly "QMH Add Message to Queue.vi"("Messages"=string[] ["emit", "405 emit", "532 emit", "660 emit"], "queue in"=w123) -> ()  [unwired: 8 in, 2 out]
      }
      event "375 Power (mW)": Value Change {
        n26 = event-data() -> ("NewVal"=w125:dbl)  [unwired: 1 in, 5 out]
        n27 = Format Into String(w125) -> (resulting string=w124:string)  [unwired: 3 in, 1 out]
        n28 = call-poly "QMH Add Message to Queue.vi"("Parameter"=w124, "Message"="532 Power", "queue in"=w126) -> ()  [unwired: 7 in, 2 out]
      }
      event "445 Power (mW)": Value Change {
        n29 = event-data() -> ("NewVal"=w129:dbl)  [unwired: 1 in, 5 out]
        n30 = Format Into String(w129) -> (resulting string=w128:string)  [unwired: 3 in, 1 out]
        n31 = call-poly "QMH Add Message to Queue.vi"("Parameter"=w128, "Message"="782 Power", "queue in"=w130) -> ()  [unwired: 7 in, 2 out]
      }
      event "getbkg": Value Change {
        n32 = event-data() -> ()  [unwired: 1 in, 6 out]
        n33 = call-poly "QMH Add Message to Queue.vi"("Message"="background", "queue in"=w132) -> ()  [unwired: 8 in, 2 out]
      }
      event "Alignment Mode": Value Change {
        n34 = event-data() -> ()  [unwired: 1 in, 6 out]
        n35 = call-poly "QMH Add Message to Queue.vi"("Message"="align", "queue in"=w134) -> ()  [unwired: 8 in, 2 out]
      }
      event "sweep": Value Change {
        n36 = event-data() -> ()  [unwired: 1 in, 6 out]
        n37 = call-poly "QMH Add Message to Queue.vi"("Message"="sweep", "queue in"=w137) -> ()  [unwired: 8 in, 2 out]
      }
      event "set freqs": Value Change {
        n38 = event-data() -> ()  [unwired: 1 in, 6 out]
        n39 = local read "Calculated Resonance (Hz)"() -> (w140:dbl)
        n40 = Format Into String(w140) -> (resulting string=w139:string, error out=w138:errorcluster)  [unwired: 3 in]
        n41 = call-poly "QMH Add Message to Queue.vi"("error in (no error)"=w138, "Parameter"=w139, "Message"="setfreqs", "queue in"=w141) -> ()  [unwired: 6 in, 2 out]
      }
      event "Save Data": Value Change {
        n42 = event-data() -> ("NewVal"=w145:bool)  [unwired: 1 in, 5 out]
        n43 = Format Into String(w145) -> (resulting string=w144:string, error out=w143:errorcluster)  [unwired: 3 in]
        n44 = call-poly "QMH Add Message to Queue.vi"("error in (no error)"=w143, "Parameter"=w144, "Message"="namefiles", "queue in"=w146) -> ()  [unwired: 6 in, 2 out]
      }
      event "Switch Filter": Value Change {
        n45 = event-data() -> ("NewVal"=w150:bool)  [unwired: 1 in, 5 out]
        n46 = local write "Filtering"(w150) -> ()
        n47 = Format Into String(w150) -> (resulting string=w148:string)  [unwired: 3 in, 1 out]
        n48 = call-poly "QMH Add Message to Queue.vi"("Parameter"=w148, "Message"="filterswitch", "queue in"=w151) -> ()  [unwired: 7 in, 2 out]
      }
      event "Time has Elapsed": Value Change {
        n49 = event-data() -> ("NewVal"=w154:bool)  [unwired: 1 in, 5 out]
        n50 = local read "Filtering"() -> (w153:bool)
        n51 = call "filterCreateMsg.vi"("time elapsed?"=w154, "auto sweep (true)"="Autosweep?", "filtering (true)"=w153, "queue in"=w155) -> ()  [unwired: 6 in, 2 out]
      }
      event "Calculated Resonance (Hz)": Value Change {
        n52 = event-data() -> ("NewVal"=w158:dbl)  [unwired: 1 in, 5 out]
        n53 = Format Into String(w158) -> (resulting string=w156:string, error out=w157:errorcluster)  [unwired: 3 in]
        n54 = call-poly "QMH Add Message to Queue.vi"("error in (no error)"=w157, "Parameter"=w156, "Message"="setfreqs", "queue in"=w160) -> ()  [unwired: 6 in, 2 out]
      }
      event "PAS Save": Value Change {
        n55 = event-data() -> ()  [unwired: 1 in, 6 out]
        n56 = call-poly "QMH Add Message to Queue.vi"("Message"="setwd", "queue in"=w162) -> ()  [unwired: 8 in, 2 out]
      }
      event "Chopper": Mouse Up {
        n57 = event-data() -> ()  [unwired: 1 in, 8 out]
        n58 = call-poly "QMH Add Message to Queue.vi"("Message"="chopper enable", "queue in"=w164) -> ()  [unwired: 8 in, 2 out]
      }
      event "save spectrum": Mouse Up {
        n59 = event-data() -> ()  [unwired: 1 in, 8 out]
        n60 = call-poly "QMH Add Message to Queue.vi"("Message"="savespec", "queue in"=w166) -> ()  [unwired: 8 in, 2 out]
      }
    }
  }
  n61 = call <userlib>:"WaveIO_Open.vi"("idev"="mic id", "Watchdog timeout (msec) (default=OFF)"=2000, "device type (Record)"=w53, "Buffer Config"=w52, "Format (44kHz, 16Bit, stereo)"=w51) -> ("Sound Handle Out"=w77:T9, "error out"=w76:errorcluster)  [unwired: 2 in]
  n62 = call <userlib>:"WaveIO_Open.vi"("idev"="pd id", "Watchdog timeout (msec) (default=OFF)"=2000, "device type (Record)"=w53, "Buffer Config"=w52, "Format (44kHz, 16Bit, stereo)"=w51) -> ("Sound Handle Out"=w61:T9, "error out"=w62:errorcluster)  [unwired: 2 in]
  n63 = Obtain Queue(element data type="Data 2") -> (queue out=w45:refnum<queue>, error out=w84:errorcluster)  [unwired: 4 in, 1 out]
  n64 = Obtain Queue(element data type="Data 2") -> (queue out=w49:refnum<queue>, error out=w58:errorcluster)  [unwired: 4 in, 1 out]
  n65 = call "picoSetChannel.vi"("error in (no error)"=w7, "Channel B Settings"="Channel B Settings", "Channel A Settings"="Channel A Settings", "Handle Out"=w6) -> ("error out"=w18:errorcluster, "Handle Out"=w21:i16)  [unwired: 6 in]
  n66 = call <userlib>:"WaveIO_Start.vi"("error in (no error)"=w76, "Handle"=w77) -> ("error out"=w74:errorcluster, "Handle Out"=w75:T9)
  n67 = call <userlib>:"WaveIO_Start.vi"("error in (no error)"=w62, "Handle"=w61) -> ("error out"=w64:errorcluster, "Handle Out"=w63:T9)
  n68 = call "picoGetTimebase.vi"("error in (no error)"=w18, "Rapid Block Acquisition Settings"="Rapid Block Acquisition Settings", "handle in"=w21) -> ("error out"=w19:errorcluster, "Sample Interval"=w25:sgl, "handle out"=w20:i16)  [unwired: 6 in]
  n69 = while {
    shift-right: [w175] -> w85
    shift-left: w45 -> [w173]
    shift-right: [w176] -> w86
    shift-left: w84 -> [w174]
    tunnel: w75 -> [w171]
    tunnel: w74 -> [w170]
    tunnel: [w168] -> w71
    tunnel: [w167] -> w70
    stop <- w172 stop-if-true
    # "Microphone DAQ Loop (Producer)"
    n70 = call <userlib>:"WaveIO_Record.vi"("Handle"=w171, "error in (no error)"=w170) -> ("Handle Out"=w168:T9, "Data"=w169:i32[][], "error out"=w167:errorcluster)  [unwired: 1 in, 2 out]
    n71 = local read "Exit"() -> (w172:bool)
    n72 = Enqueue Element(queue=w173, element=w169, error in (no error)=w174) -> (queue out=w175:refnum<queue>, error out=w176:errorcluster)  [unwired: 1 in, 1 out]
  }
  n73 = while {
    shift-right: [w185] -> w57
    shift-left: w49 -> [w183]
    shift-right: [w186] -> w56
    shift-left: w58 -> [w184]
    tunnel: w63 -> [w181]
    tunnel: w64 -> [w180]
    tunnel: [w178] -> w67
    tunnel: [w177] -> w68
    stop <- w182 stop-if-true
    # "PD DAQ Loop (Producer)"
    n74 = call <userlib>:"WaveIO_Record.vi"("Handle"=w181, "error in (no error)"=w180) -> ("Handle Out"=w178:T9, "Data"=w179:i32[][], "error out"=w177:errorcluster)  [unwired: 1 in, 2 out]
    n75 = local read "Exit"() -> (w182:bool)
    n76 = Enqueue Element(queue=w183, element=w179, error in (no error)=w184) -> (queue out=w185:refnum<queue>, error out=w186:errorcluster)  [unwired: 1 in, 1 out]
  }
  n77 = call "picoTrigger.vi"("Trigger Channel Settings"="Channel B Settings", "error in (no error)"=w19, "maxADC"=w26, "Trigger Settings"="Trigger Settings", "Handle In"=w20) -> ("error out"=w12:errorcluster, "Range"=w27:u16, "handle out"=w13:i16)  [unwired: 4 in]
  n78 = Obtain Queue(element data type=i16[][] [] ("buffer")) -> (queue out=w3:refnum<queue>, error out=w31:errorcluster)  [unwired: 4 in, 1 out]
  n79 = call "picoSetMem.vi"("error in (no error)"=w12, "Rapid Block Acquisition Settings"="Rapid Block Acquisition Settings", "Handle In"=w13) -> ("timebase"=w10:u32, "postTriggerSamples"=w9:u32, "Handle Out"=w8:i16, "nCaptures"=w11:u16)  [unwired: 4 in, 1 out]
  n80 = call "picoExtractSettings.vi"("Rapid Block Acquisition Settings"="Rapid Block Acquisition Settings") -> ("Down-Sample Mode"=w17:i32, "Down Sample Ratio"=w16:u32, "Numeric"=w15:i32)  [unwired: 8 in]
  n81 = while {
    tunnel: w8 -> [w204]
    tunnel: w9 -> [w203]
    tunnel: w10 -> [w202]
    tunnel: w11 -> [w208]
    tunnel: w15 -> [w200]
    tunnel: w16 -> [w199]
    tunnel: w17 -> [w198]
    tunnel: [w193] -> w30
    shift-right: [w190] -> _
    shift-left: w3 -> [w191]
    shift-right: [w188] -> w4
    shift-left: w31 -> [w187]
    stop <- w197 stop-if-true
    # "CRD Acquisition Loop (Producer)"
    n82 = call "picoRunBlock.vi"("error in (no error)"=w187, "timebase"=w202, "postTriggerSamples"=w203, "Handle In"=w204) -> ("error out"=w207:errorcluster, "handle"=w206:i16)  [unwired: 5 in, 1 out]
    n83 = call "picoReady.vi"("error in (no error)"=w207, "handle in"=w206) -> ("error out"=w205:errorcluster, "handle out"=w201:i16)  [unwired: 8 in]
    n84 = call "picoGetValues.vi"("Down-Sample Mode"=w198, "Down Sample Ratio"=w199, "nCaptures"=w208, "error in (no error)"=w205, "postTriggerSamples"=w200, "Handle In"=w201) -> ("error out"=w189:errorcluster, "buffer"=w192:i16[][], "handle"=w193:i16)  [unwired: 3 in]
    n85 = local read "Exit"() -> (w195:bool)
    n86 = Enqueue Element(queue=w191, element=w192, error in (no error)=w189) -> (queue out=w190:refnum<queue>, error out=w188:errorcluster)  [unwired: 1 in, 1 out]
    n87 = Unbundle By Name(w188) -> ("status"=w196:bool)
    n88 = Or(x=w196, y=w195) -> (x .or. y?=w197:bool)
    n89 = Wait (ms)(milliseconds to wait="crd delay") -> ()  [unwired: 1 out]
  }
  "error out" <- w4
  n90 = call <userlib>:"WaveIO_Stop.vi"("error in (no error)"=w70, "Handle"=w71) -> ("error out"=w72:errorcluster, "Handle Out"=w73:T9)
  n91 = Release Queue(queue=w85, error in (no error)=w86) -> (error out=w82:errorcluster)  [unwired: 1 in, 2 out]
  n92 = call <userlib>:"WaveIO_Stop.vi"("error in (no error)"=w68, "Handle"=w67) -> ("error out"=w66:errorcluster, "Handle Out"=w65:T9)
  n93 = Release Queue(queue=w57, error in (no error)=w56) -> (error out=w55:errorcluster)  [unwired: 1 in, 2 out]
  n94 = call <userlib>:"WaveIO_Close.vi"("error in (no error)"=w72, "Handle"=w73) -> ("error out"=w69:errorcluster)  [unwired: 1 out]
  n95 = call <userlib>:"WaveIO_Close.vi"("error in (no error)"=w66, "Handle"=w65) -> ("error out"=w54:errorcluster)  [unwired: 1 out]
  n96 = Divide(x=1.0, y=44100.0) -> (x/y=w46:dbl)
  n97 = Merge Errors(w69, w82, w54, w55) -> (w81:errorcluster)
  n98 = Obtain Queue(element data type=cluster{dbl, dbl, dbl} {0.0, 0.0, 0.0}) -> (queue out=w34:refnum<queue>, error out=w39:errorcluster)  [unwired: 4 in, 1 out]
  n99 = Obtain Queue(element data type=cluster{dbl, dbl, dbl} {0.0, 0.0, 0.0}) -> (queue out=w33:refnum<queue>, error out=w42:errorcluster)  [unwired: 4 in, 1 out]
  n100 = while "Message Processor" {
    shift-left: w95 -> [w223]
    shift-right: [w215] -> w91
    tunnel: w80 -> [w222]
    shift-left: "State Variables" -> [w228]
    shift-right: [w227] -> _
    tunnel: "320 Port" -> [w219]
    tunnel: "375 Port" -> [w218]
    tunnel: "445 Port" -> [w217]
    tunnel: "Teensy Port" -> [w216]
    shift-right: [w213] -> _
    shift-left: _ -> [w212]
    tunnel: w32 -> [w210]
    tunnel: "Chopper Port" -> [w209]
    stop <- w226 stop-if-true
    w220 = 100  # Timeout
    n101 = call "QMH Get Next Message from Queue.vi"("error in (no error)"=w223, "ms timeout (1)"=w220, "queue in"=w222) -> ("error out"=w224:errorcluster, "Next Parameter"=w211:string, "Next Message"=w221:string, "queue out"=w225:refnum<queue>, "Stop QMH"=w226:bool)  [unwired: 3 in]
    n102 = case shown="Default" w221 {
      selector: w221 -> [_ w257 _ _ _ _ _ _ _ _ _ _ _ _ _ _ _ _ _ _ _]
      tunnel: [w253 w258 w276 w295 w352 w375 w413 w442 w448 w454 w461 w468 w475 w495 w502 w526 w538 w554 w597 w603 w616] -> w227
      tunnel: w228 -> [w253 w258 w276 w295 w352 w375 w413 w442 w448 w454 w461 w468 w475 w495 w502 w526 w538 w554 w597 w603 w616]
      tunnel: w225 -> [_ _ _ w288 _ _ _ _ _ _ _ _ _ _ _ _ _ _ _ w601 w617]
      tunnel: w224 -> [w246 w254 w264 w294 w350 w370 w410 w444 w450 w452 w458 w465 w473 w496 w499 w524 w537 w555 w594 w602 w618]
      tunnel: [w245 w254 w260 w287 w349 w372 w411 w440 w446 w452 w459 w466 w469 w496 w498 w523 w537 w555 w595 w599 w604] -> w215
      tunnel: w219 -> [w243 _ w275 w286 _ _ w412 _ _ _ _ _ w472 _ _ _ _ _ _ _ w613]
      tunnel: w218 -> [w241 _ w273 w290 _ _ _ w441 _ _ w460 _ w471 _ _ _ _ _ _ _ w612]
      tunnel: w217 -> [w242 _ w272 w293 _ _ _ _ w447 _ _ w467 w470 _ _ _ _ _ _ _ w611]
      tunnel: w216 -> [_ _ w270 w289 w351 w373 _ _ _ _ _ _ _ _ w500 w525 _ _ _ _ w614]
      tunnel: w211 -> [_ _ _ _ w348 w368 _ _ _ _ w455 w462 _ _ _ w522 w536 _ _ _ _]
      tunnel: w210 -> [_ _ _ _ _ _ _ _ _ _ _ _ _ _ _ _ w535 _ _ _ _]
      tunnel: w209 -> [_ _ w265 _ _ _ w408 _ _ _ _ _ _ _ _ _ _ _ w596 _ w606]
      frame "", "Wait" {
        # "Update the front panel"
        # "Idle Case - this case is called after a Timeout on the Get Next Message from Queue VI, if no new messages are present on the queue. This case can be used for housekeeping tasks such as updating the UI."
        n103 = Get Date/Time String(want seconds? (F)=TRUE) -> (date string=w252:string, time string=w251:string)  [unwired: 2 in]
        n104 = call-poly "laserDiagnose.vi"("320 Port"=w243, "375 Port in"=w241, "445 Port 3"=w242, "error in (no error)"=w246) -> ("Powers"=→"Laser Powers":T10, "Currents"=→"Laser Currents":T11, "Temperatures"=→"Laser Temperatures":T2, "Overtemp"=→"Overtemp":bool, "error out"=w245:errorcluster)  [unwired: 7 in]
        n105 = Concatenate Strings(w252, " " ("string"), w251) -> (→"Status":string)
      }
      frame Default {
        # "Call this case if a message is received that is not handled \nby any other case. Typically this is a programming error\nas a result of a typo or unhandled message/missing message handler."
        n106 = Format Into String(format string="DevError: Missing message handler for '%s\" message." ("message"), w257) -> (resulting string=w255:string)  [unwired: 2 in, 1 out]
        n107 = One Button Dialog(message=w255) -> ()  [unwired: 1 in, 1 out]
      }
      frame "Initialize" {
        w266 = u32 115200 ("baud rate (9600)")
        # "Initialize the state variables and user interface\nInitialize serial connections"
        n108 = call-poly "VISA Configure Serial Port"("VISA resource name"=w265, "baud rate (9600)"=w266, "error in (no error)"=w264) -> ("VISA resource name out"=w263:refnum<visa-resource-name>, "error out"=w262:errorcluster)  [unwired: 11 in]
        n109 = disable-structure shown="Disabled" {
          disable-tunnel: w275 -> [w285 _]
          disable-tunnel: [w284 _] -> w274
          disable-tunnel: w262 -> [w283 _]
          disable-tunnel: u32 19200 ("baud rate (9600)") -> [w282 _]
          frame Disabled {
            n110 = call-poly "VISA Configure Serial Port"("VISA resource name"=w285, "baud rate (9600)"=w282, "error in (no error)"=w283) -> ("error out"=w284:errorcluster)  [unwired: 11 in, 1 out]
          }
          frame Enabled {
          }
        }
        n111 = call-poly "VISA Configure Serial Port"("VISA resource name"=w273, "baud rate (9600)"=w266, "error in (no error)"=w274) -> ("error out"=w271:errorcluster)  [unwired: 11 in, 1 out]
        n112 = call-poly "VISA Configure Serial Port"("VISA resource name"=w272, "baud rate (9600)"=w266, "error in (no error)"=w271) -> ("error out"=w269:errorcluster)  [unwired: 11 in, 1 out]
        n113 = call-poly "VISA Configure Serial Port"("VISA resource name"=w270, "error in (no error)"=w269) -> ("VISA resource name out"=w268:refnum<visa-resource-name>, "error out"=w267:errorcluster)  [unwired: 12 in]
        n114 = property class="Instr" props=["Baud"](reference=w268, error in=w267) -> (error out=w261:errorcluster)  [unwired: 2 out]
        n115 = disable-structure shown="Disabled" {
          disable-tunnel: w263 -> [w281 _]
          disable-tunnel: w261 -> [w280 _]
          disable-tunnel: [w279 _] -> w260
          frame Disabled {
            w278 = u16 1 items=["stop", "start"] ("start/stop")
            n116 = call "chopperStartStop.vi"("error in (no error)"=w280, "start/stop"=w278, "VISA Refnum in"=w281) -> ("error out"=w279:errorcluster, "Chopper On?"=w277:bool)  [unwired: 6 in, 1 out]
            n117 = local write "Chopper On"(w277) -> ()
          }
          frame Enabled {
          }
        }
      }
      frame "sweep" {
        # "Perform a frequency sweep and calculate the resonance frequency"
        n118 = stacked-sequence {
          seq-local: [_ w308 _ _] -> [_ _ w336 _]
          tunnel: w294 -> [w297 w302 _ _]
          tunnel: "Data End Frequency (Hz)" -> [_ w305 w330 _]
          tunnel: "Data Start Frequency (Hz)" -> [_ w304 w329 _]
          tunnel: w293 -> [_ _ _ _]
          tunnel: w290 -> [w298 _ _ w343]
          tunnel: w289 -> [_ w303 _ _]
          tunnel: w288 -> [_ _ _ w346]
          tunnel: [w296 _ _ _] -> w287
          tunnel: w286 -> [_ _ _ _]
          frame #0 {
            # "Turn UV lasers off for scan."
            n119 = call "laserOnOff.vi"("error in (no error)"=w297, "Emission (F = OFF)"=FALSE, "VISA Refnum in"=w298) -> ("error out"=w296:errorcluster)  [unwired: 6 in, 2 out]
            n120 = Wait (ms)(milliseconds to wait=u32 5000) -> ()  [unwired: 1 out]
            n121 = local write "Status"("Conducting Frequency Sweep" ("Status")) -> ()
          }
          frame #1 {
            n122 = Subtract(x=w305, y=w304) -> (x-y=w306:i32)
            n123 = for {
              N: w306 -> [w312]
              tunnel: [w317] -> w308 mode=indexing
              tunnel: w304 -> [w316]
              tunnel: w305 -> [w315]
              tunnel: w302 -> [_]
              i -> [w309]
              # "Get microphone data."
              # "Listen for N*2000\n seconds"
              n124 = Increment(x=w309) -> (x+1=w310:i32)
              n125 = Divide(x=w310, y=w312) -> (x/y=→"sweep progress":dbl)
              n126 = local read "micfft"() -> (w314:cluster{"f0":dbl, "df":dbl, "magnitude":dbl[]})
              n127 = Unbundle By Name(w314) -> ("magnitude"=w313:dbl[])
              n128 = Wait (ms)(milliseconds to wait=u32 2000) -> ()  [unwired: 1 out]
              n129 = call "fftGetMax.vi"("End Frequency (Hz)"=w315, "Start Frequency (Hz)"=w316, "Magnitudes"=w313) -> ("max value"=w317:dbl)  [unwired: 8 in]
            }
            n130 = case shown="True" TRUE ("sweep?") {
              tunnel: w304 -> [_ w324]
              tunnel: w305 -> [_ w323]
              tunnel: w303 -> [_ w322]
              tunnel: [w319 w321] -> _
              tunnel: w302 -> [w319 w320]
              frame False {
              }
              frame True {
                # "Scan laser freq.\nwith Teensy"
                n131 = call "teensySweepFreq.vi"("error in (no error)"=w320, "end f, Hz (1385)"=w323, "start f, Hz (1355)"=w324, "VISA Refnum in"=w322) -> ("error out"=w321:errorcluster)  [unwired: 7 in]
              }
            }
          }
          frame #2 {
            # "Calculate resonance frequency;\ndisplay and save scan."
            n132 = Wait (ms)(milliseconds to wait=u32 5000) -> ()  [unwired: 1 out]
            n133 = local read "PAS Save"() -> (w325:bool)
            n134 = To Double Precision Float(number=w330) -> (double precision float=w327:dbl)
            n135 = To Double Precision Float(number=w329) -> (double precision float=w328:dbl)
            n136 = call "resCalc.vi"("Frequency Sweep"=w336, "Start F, Hz (1355)"=w329) -> ("F-res, Hz"=w334:dbl, "Frequency Scan"=w326:cluster{i32[], "Best Gaussian Fit":dbl[]}[])  [unwired: 8 in]
            "freqscan" <- w326
            n137 = In Range and Coerce(upper limit=w327, x=w334, lower limit=w328) -> (In Range?=w333:bool)  [unwired: 1 out]
            n138 = case shown="True" w325 {
              tunnel: w326 -> [_ w340]
              tunnel: w334 -> [_ w339]
              frame False {
              }
              frame True {
                n139 = local read "sweeps"() -> (w338:path)
                n140 = call "saveFreqSweep.vi"("f-res, Hz"=w339, "Frequency Scan"=w340, "file path (dialog if empty)"=w338) -> ()  [unwired: 9 in]
              }
            }
            n141 = And(x=w333, y=TRUE ("check freqs?")) -> (x .and. y?=w331:bool)
            n142 = case shown="True" w331 {
              tunnel: w334 -> [_ w337]
              frame False {
              }
              frame True {
                n143 = property on="Calculated Resonance (Hz)" class="DigNum (strict)"("Val(Sgnl)"=w337) -> ()  [unwired: 2 in, 2 out]
                "Calculated Resonance (Hz)" <- w337
              }
            }
          }
          frame #3 {
            # "Turn UV lasers back on."
            n144 = local read "375 Power (mW)"() -> (w342:dbl)
            n145 = call "laserOnOff.vi"("Emission (F = OFF)"=TRUE, "Power, mW (100)"=w342, "VISA Refnum in"=w343) -> ("error out"=w341:errorcluster)  [unwired: 6 in, 2 out]
            n146 = call-poly "QMH Add Message to Queue.vi"("error in (no error)"=w341, "Parameter"="532 F (Hz)", "Message"="freqset", "queue in"=w346) -> ()  [unwired: 6 in, 2 out]
          }
        }
      }
      frame "freqset" {
        # "Set the frequency of the Teensy's modulation\nsignal for single laser (if single frequency is changed)."
        # "Set the laser frequency.  Case for \"red\", \"blue\", or \"green\"."
        n147 = case shown="\"375 F (Hz)\"" w348 {
          tunnel: w350 -> [w357 w362 w367]
          tunnel: [w356 w361 w366] -> w349
          tunnel: w351 -> [w353 w358 w364]
          frame "320 F (Hz) ", Default {
            w355 = u16 0 items=["blue", "green", "red"] ("laser")
            n148 = call "freqSet.vi"("error in (no error)"=w357, "laser"=w355, "Freq, Hz (1370)"="320 F (Hz)", "Teensy Port"=w353) -> ("error out"=w356:errorcluster)  [unwired: 6 in, 1 out]
          }
          frame "375 F (Hz)" {
            w360 = u16 1 items=["blue", "green", "red"] ("laser")
            n149 = call "freqSet.vi"("error in (no error)"=w362, "laser"=w360, "Freq, Hz (1370)"="375 F (Hz)", "Teensy Port"=w358) -> ("error out"=w361:errorcluster)  [unwired: 6 in, 1 out]
          }
          frame "445 F (Hz)" {
            w363 = u16 2 items=["blue", "green", "red", "ir"] ("laser")
            n150 = call "freqSet.vi"("error in (no error)"=w367, "laser"=w363, "Freq, Hz (1370)"="445 F (Hz)", "Teensy Port"=w364) -> ("error out"=w366:errorcluster)  [unwired: 6 in, 1 out]
          }
        }
      }
      frame "setfreqs" {
        # "Set the frequency of the Teensy's modulation\nsignal for all lasers at once."
        # "Set laser frequencies to resonance frequency calculated in sweep."
        n151 = Scan From String(input string=w368, error in=w370) -> (error out=w369:errorcluster, output 1=w371:dbl)  [unwired: 3 in, 2 out]
        n152 = for {
          N: 3 -> [_]
          tunnel: [w381] -> w372
          tunnel: w369 -> [w380]
          tunnel: w373 -> [w377]
          tunnel: w371 -> [w379]
          i -> [w378]
          n153 = flat-sequence {
            tunnel: w377 -> [w382]
            tunnel: [w382] -> w376
            frame #0 {
              n154 = Wait (ms)(milliseconds to wait=u32 1000) -> ()  [unwired: 1 out]
            }
          }
          n155 = case shown="0" w378 {
            tunnel: [w389 w397 w405] -> w381
            tunnel: w380 -> [w387 w394 w402]
            tunnel: w376 -> [w386 w393 w401]
            tunnel: w379 -> [w384 w390 w398]
            frame 0 {
              w388 = u16 2 items=["blue", "green", "red"] ("laser")
              n156 = To Long Integer(number=w384) -> (32bit integer=w385:i32)
              n157 = local write "445 F (Hz)"(w385) -> ()
              n158 = call "freqSet.vi"("error in (no error)"=w387, "laser"=w388, "Freq, Hz (1370)"=w385, "Teensy Port"=w386) -> ("error out"=w389:errorcluster)  [unwired: 6 in, 1 out]
            }
            frame 1, Default {
              w396 = u16 1 items=["blue", "green", "red"] ("laser")
              n159 = Add(x=w390, y=2.0) -> (x+y=w392:dbl)
              n160 = To Long Integer(number=w392) -> (32bit integer=w391:i32)
              n161 = call "freqSet.vi"("error in (no error)"=w394, "laser"=w396, "Freq, Hz (1370)"=w391, "Teensy Port"=w393) -> ("error out"=w397:errorcluster)  [unwired: 6 in, 1 out]
              n162 = local write "375 F (Hz)"(w391) -> ()
            }
            frame 2 {
              w404 = u16 0 items=["blue", "green", "red"] ("laser")
              n163 = Subtract(x=w398, y=2.0) -> (x-y=w400:dbl)
              n164 = To Long Integer(number=w400) -> (32bit integer=w399:i32)
              n165 = call "freqSet.vi"("error in (no error)"=w402, "laser"=w404, "Freq, Hz (1370)"=w399, "Teensy Port"=w401) -> ("error out"=w405:errorcluster)  [unwired: 6 in, 1 out]
              n166 = local write "320 F (Hz)"(w399) -> ()
            }
          }
        }
      }
      frame "320 emit" {
        w409 = u16 2 items=["stop", "start", "ask"] ("start/stop")
        n167 = call "chopperStartStop.vi"("error in (no error)"=w410, "start/stop"=w409, "VISA Refnum in"=w408) -> ("error out"=w406:errorcluster, "Chopper On?"=w407:bool)  [unwired: 6 in, 1 out]
        n168 = case shown="True" w407 {
          tunnel: w412 -> [_ w419]
          tunnel: [w415 w418] -> w411
          tunnel: w406 -> [w415 w416]
          frame False {
            n169 = One Button Dialog(message="Turn on chopper first!") -> ()  [unwired: 1 in, 1 out]
          }
          frame True {
            # "Turn laser on or off"
            n170 = case shown="True" "320 Emission" {
              tunnel: [w424 w432] -> w418
              tunnel: [w425 w433] -> _
              tunnel: w419 -> [w421 w430]
              tunnel: w416 -> [w420 w431]
              frame False {
                n171 = VISA Write(VISA resource name=w421, write buffer="22891\t3\t1030\r", error in (no error)=w420) -> (VISA resource name out=w422:refnum<visa-resource-name>, error out=w423:errorcluster)  [unwired: 1 out]
                n172 = property class="Instr"(reference=w422, error in=w423) -> (reference out=w426:refnum<visa-resource-name>, error out=w427:errorcluster, "Bytes at Port"=w428:u32)
                n173 = VISA Read(VISA resource name=w426, byte count=w428, error in (no error)=w427) -> (VISA resource name out=w425:refnum<visa-resource-name>, error out=w424:errorcluster)  [unwired: 2 out]
              }
              frame True {
                n174 = VISA Write(VISA resource name=w430, write buffer="22891\t3\t1020\r", error in (no error)=w431) -> (VISA resource name out=w435:refnum<visa-resource-name>, error out=w434:errorcluster)  [unwired: 1 out]
                n175 = property class="Instr"(reference=w435, error in=w434) -> (reference out=w438:refnum<visa-resource-name>, error out=w437:errorcluster, "Bytes at Port"=w436:u32)
                n176 = VISA Read(VISA resource name=w438, byte count=w436, error in (no error)=w437) -> (VISA resource name out=w433:refnum<visa-resource-name>, error out=w432:errorcluster)  [unwired: 2 out]
              }
            }
          }
        }
      }
      frame "375 emit" {
        # "Turn laser on or off"
        n177 = call "laserOnOff.vi"("error in (no error)"=w444, "Emission (F = OFF)"="375 Emission", "Power, mW (100)"="375 Power (mW)", "VISA Refnum in"=w441) -> ("error out"=w440:errorcluster)  [unwired: 5 in, 2 out]
      }
      frame "445 emit" {
        # "Turn laser on or off"
        n178 = call "laserOnOff.vi"("error in (no error)"=w450, "Emission (F = OFF)"="445 Emission", "Power, mW (100)"="445 Power (mW)", "VISA Refnum in"=w447) -> ("error out"=w446:errorcluster)  [unwired: 5 in, 2 out]
      }
      frame "emit" {
        # "Turn on all lasers."
        n179 = local write "320 Emission"("All Emit") -> ()
        n180 = local write "375 Emission"("All Emit") -> ()
        n181 = local write "445 Emission"("All Emit") -> ()
      }
      frame "532 Power" {
        n182 = Scan From String(input string=w455, error in=w458) -> (error out=w457:errorcluster, output 1=w456:dbl)  [unwired: 3 in, 2 out]
        n183 = call "laserSetPower.vi"("error in (no error)"=w457, "Laser Power (mW)"=w456, "VISA Refnum in"=w460) -> ("error out"=w459:errorcluster)  [unwired: 7 in, 1 out]
      }
      frame "782 Power" {
        n184 = Scan From String(input string=w462, error in=w465) -> (error out=w464:errorcluster, output 1=w463:dbl)  [unwired: 3 in, 2 out]
        n185 = call "laserSetPower.vi"("error in (no error)"=w464, "Laser Power (mW)"=w463, "VISA Refnum in"=w467) -> ("error out"=w466:errorcluster)  [unwired: 7 in, 1 out]
      }
      frame "align" {
        # "Set power of all lasers to 5 mW for alignment"
        n186 = case shown="False" "Alignment Mode" {
          tunnel: w473 -> [w483 w492]
          tunnel: w472 -> [w482 w491]
          tunnel: w471 -> [w481 w490]
          tunnel: w470 -> [w480 w489]
          tunnel: [w477 w486] -> w469
          frame True {
            w476 = 5.0 ("Laser Power (mW)")
            n187 = call "laserSetPower.vi"("error in (no error)"=w483, "Laser Power (mW)"=w476, "VISA Refnum in"=w482) -> ("error out"=w479:errorcluster)  [unwired: 7 in, 1 out]
            n188 = call "laserSetPower.vi"("error in (no error)"=w479, "Laser Power (mW)"=w476, "VISA Refnum in"=w481) -> ("error out"=w478:errorcluster)  [unwired: 7 in, 1 out]
            n189 = call "laserSetPower.vi"("error in (no error)"=w478, "Laser Power (mW)"=w476, "VISA Refnum in"=w480) -> ("error out"=w477:errorcluster)  [unwired: 7 in, 1 out]
          }
          frame False, Default {
            n190 = local read "375 Power (mW)"() -> (w485:dbl)
            n191 = local read "445 Power (mW)"() -> (w484:dbl)
            n192 = call "laserSetPower.vi"("error in (no error)"=w492, "VISA Refnum in"=w491) -> ("error out"=w488:errorcluster)  [unwired: 8 in, 1 out]
            n193 = call "laserSetPower.vi"("error in (no error)"=w488, "Laser Power (mW)"=w485, "VISA Refnum in"=w490) -> ("error out"=w487:errorcluster)  [unwired: 7 in, 1 out]
            n194 = call "laserSetPower.vi"("error in (no error)"=w487, "Laser Power (mW)"=w484, "VISA Refnum in"=w489) -> ("error out"=w486:errorcluster)  [unwired: 7 in, 1 out]
          }
        }
      }
      frame "background" {
        n195 = local read "mic ts"() -> (w494:T7)
        n196 = local read "tau"() -> (w493:dbl)
        n197 = local write "Bkg Values (mV)"(w494) -> ()
        n198 = local write "tau0"(w493) -> ()
      }
      frame "filter" {
        n199 = local read "Filtering"() -> (w501:bool)
        n200 = case shown="True" w501 {
          tunnel: w500 -> [w505 w514]
          tunnel: w499 -> [w504 w512]
          tunnel: [w503 w513] -> w498
          frame False {
            n201 = Multiply(x="Filter Length (min)", y=60.0) -> (x*y=w508:dbl)
            n202 = local write "Time Target (s)"(w508) -> ()
            n203 = VISA Write(VISA resource name=w505, write buffer="v.1", error in (no error)=w504) -> (error out=w503:errorcluster)  [unwired: 2 out]
            "Filtering" <- TRUE
          }
          frame True {
            n204 = flat-sequence {
              tunnel: w512 -> [w520]
              tunnel: [w520] -> w511
              frame #0 {
                n205 = local read "mic ts"() -> (w521:T7)
                n206 = local write "Bkg Values (mV)"(w521) -> ()
              }
            }
            n207 = local write "Filtering"(FALSE) -> ()
            n208 = VISA Write(VISA resource name=w514, write buffer="v.0", error in (no error)=w511) -> (error out=w513:errorcluster)  [unwired: 2 out]
            n209 = Multiply(x="Sample Length (min)", y=60.0) -> (x*y=w516:dbl)
            n210 = local write "Time Target (s)"(w516) -> ()
          }
        }
        n211 = Wait (ms)(milliseconds to wait=u32 500) -> ()  [unwired: 1 out]
      }
      frame "filterswitch" {
        n212 = case shown="\"TRUE\"" w522 {
          tunnel: w525 -> [w529 w534]
          tunnel: w524 -> [w528 w533]
          tunnel: [w527 w532] -> w523
          frame "FALSE", Default {
            n213 = VISA Write(VISA resource name=w529, write buffer="v.0", error in (no error)=w528) -> (error out=w527:errorcluster)  [unwired: 2 out]
          }
          frame "TRUE" {
            n214 = VISA Write(VISA resource name=w534, write buffer="v.1", error in (no error)=w533) -> (error out=w532:errorcluster)  [unwired: 2 out]
          }
        }
      }
      frame "namefiles" {
        n215 = case shown="\"TRUE\"" w536 {
          tunnel: w535 -> [_ w540]
          frame "FALSE", Default {
            n216 = local write "PAS Save"(FALSE ("PAS Save")) -> ()
          }
          frame "TRUE" {
            n217 = flat-sequence {
              tunnel: [w545] -> w543
              tunnel: [w547] -> w542
              tunnel: w543 -> [w547]
              tunnel: w542 -> [w549]
              tunnel: w541 -> [w548]
              frame #0 {
                n218 = call "saveSetDirectory.vi"() -> ("pas"=w545:path, "sweeps"=→"sweeps":path)  [unwired: 11 in, 3 out]
                "pas" <- w545
              }
              frame #1 {
                "PAS Save" <- TRUE ("PAS Save")
              }
              frame #2 {
                n219 = call-poly <vilib>:"Write To Spreadsheet File.vi"("append to file? (new file:F)"=TRUE, "2D data"=w548, "file path (dialog if empty)"=w549) -> ()  [unwired: 5 in, 1 out]
              }
            }
            n220 = Build Array(w540) -> (w541:string[][])
          }
        }
      }
      frame "savespec" {
        w551 = -1
        w587 = TRUE ("append to file? (new file:F)")
        n221 = local read "Filtering"() -> (w558:bool)
        n222 = local read "mic ts"() -> (w560:T7)
        n223 = local read "pd ts"() -> (w557:cluster{dbl, dbl, dbl})
        n224 = local read "tau"() -> (w552:dbl)
        n225 = Boolean To (0,1)(Boolean=w558) -> (0, 1=w566:i16)
        n226 = Unbundle(w560) -> ("422 Mean"=w573:dbl, "532 Mean"=w561:dbl, "785 Mean"=w562:dbl)
        n227 = Unbundle(w557) -> (w563:dbl, w564:dbl, w553:dbl)
        n228 = Format Date/Time String(time format string (%c)="%Y-%m-%d %H:%M:%S\t") -> (date/time string=w565:string)  [unwired: 2 in]
        n229 = Format Into String(w566) -> (resulting string=w567:string)  [unwired: 3 in, 1 out]
        n230 = Build Array(320, 375, 445) -> (w577:i32[])
        n231 = Build Array(w573, w561, w562) -> (w568:dbl[])
        n232 = Build Array(w563, w564, w553) -> (w556:dbl[])
        n233 = Build Array(w551, w551, w552) -> ()  [unwired: 1 out]
        n234 = Build Array(w565, w567) -> (w582:string[])
        n235 = Build Array(string[] ["wavelength_nm", "mic_mV", "PD_mW", ""]) -> (w586:string[][])
        n236 = Build Array(w577, w568, w556) -> (w571:dbl[][])
        n237 = Build Array(w582) -> (w583:string[][])
        n238 = Transpose 2D Array(2D array=w571) -> (transposed array=w572:dbl[][])
        n239 = Array To Spreadsheet String(array=w572, 3:"%.4e") -> (spreadsheet string=w578:string)  [unwired: 1 in]
        n240 = call-poly <vilib>:"Write To Spreadsheet File.vi"("transpose? (no:F)"=TRUE, "append to file? (new file:F)"=w587, "2D data"=w583) -> ("new file path (Not A Path if cancelled)"=w585:path)  [unwired: 5 in]
        n241 = Build Array(w578) -> (w589:string[])
        n242 = call-poly <vilib>:"Write To Spreadsheet File.vi"("transpose? (no:F)"=FALSE, "append to file? (new file:F)"=w587, "2D data"=w586, "file path (dialog if empty)"=w585) -> ("new file path (Not A Path if cancelled)"=w588:path)  [unwired: 4 in]
        n243 = call-poly <vilib>:"Write To Spreadsheet File.vi"("delimiter (\\t)"="" ("delimiter (\\t)"), "transpose? (no:F)"=FALSE, "append to file? (new file:F)"=TRUE, "1D data"=w589, "file path (dialog if empty)"=w588) -> ()  [unwired: 3 in, 1 out]
      }
      frame "chopper enable" {
        n244 = Boolean To (0,1)(Boolean="Chopper") -> (0, 1=w592:i16)
        n245 = call "chopperStartStop.vi"("error in (no error)"=w594, "start/stop"=w592, "VISA Refnum in"=w596) -> ("error out"=w595:errorcluster, "Chopper On?"=→"Chopper On":bool)  [unwired: 6 in, 1 out]
      }
      frame "Error" {
        (unwired) errorcluster {"status"=FALSE, "code"=0, "source"=""} ("error out")
        # "Proceed to Exit - remove if this is\nnot appropriate for the General Error case"
        # "General Error Case - this case is called if an error is passed using the error cluster below. Typically most new errors should be handed in each individual case and not passed in the rror cluster. If necessary a custom error handler case should be added and called from other cases."
        n246 = call <vilib>:"Simple Error Handler.vi"("error in (no error)"=w602) -> ("error out"=w598:errorcluster)  [unwired: 4 in, 4 out]
        n247 = call-poly "QMH Add Message to Queue.vi"("error in (no error)"=w598, "Message"="Exit", "queue in"=w601) -> ("error out"=w599:errorcluster)  [unwired: 7 in, 1 out]
      }
      frame "Exit" {
        # "Perform cleanup tasks: Close serial connections and clear front panel."
        n248 = call "QMH Destroy Queue.vi"("error in (no error)"=w618, "queue in"=w617) -> ("error out"=w610:errorcluster)  [unwired: 7 in, 2 out]
        n249 = for {
          N: 3 -> [_]
          tunnel: w613 -> [w632]
          tunnel: w612 -> [w630]
          tunnel: w611 -> [w629]
          tunnel: w610 -> [w628]
          tunnel: FALSE -> [w627]
          tunnel: [w626] -> w607
          i -> [w631]
          # "Close laser serial connections."
          n250 = case shown="0, Default" w631 {
            tunnel: [w639 w644 w649] -> w634
            tunnel: [w638 w643 w648] -> w633
            tunnel: w632 -> [w637 _ _]
            tunnel: w630 -> [_ w642 _]
            tunnel: w629 -> [_ _ w646]
            tunnel: w628 -> [w636 w641 w647]
            tunnel: w627 -> [w635 w640 w645]
            frame 0, Default {
              n251 = call "laserOnOff.vi"("error in (no error)"=w636, "Emission (F = OFF)"=w635, "VISA Refnum in"=w637) -> ("error out"=w639:errorcluster, "VISA Refnum out"=w638:refnum<visa-resource-name>)  [unwired: 6 in, 1 out]
              n252 = local write "320 Emission"(w635) -> ()
            }
            frame 1 {
              n253 = call "laserOnOff.vi"("error in (no error)"=w641, "Emission (F = OFF)"=w640, "VISA Refnum in"=w642) -> ("error out"=w644:errorcluster, "VISA Refnum out"=w643:refnum<visa-resource-name>)  [unwired: 6 in, 1 out]
              n254 = local write "375 Emission"(w640) -> ()
            }
            frame 2 {
              n255 = call "laserOnOff.vi"("error in (no error)"=w647, "Emission (F = OFF)"=w645, "VISA Refnum in"=w646) -> ("error out"=w649:errorcluster, "VISA Refnum out"=w648:refnum<visa-resource-name>)  [unwired: 6 in, 1 out]
              n256 = local write "445 Emission"(w645) -> ()
              n257 = local write "All Emit"(w645) -> ()
            }
          }
          n258 = VISA Close(VISA resource name=w633, error in (no error)=w634) -> (error out=w626:errorcluster)
        }
        n259 = local write "Status"("" ("Status")) -> ()
        n260 = VISA Close(VISA resource name=w614, error in (no error)=w607) -> (error out=w605:errorcluster)
        n261 = disable-structure shown="Disabled" {
          disable-tunnel: w606 -> [w625 _]
          disable-tunnel: w605 -> [w623 _]
          disable-tunnel: [w619 _] -> w604
          frame Disabled {
            w624 = u16 0 items=["stop", "start", "ask"] ("start/stop")
            n262 = call "chopperStartStop.vi"("error in (no error)"=w623, "start/stop"=w624, "VISA Refnum in"=w625) -> ("error out"=w622:errorcluster, "Chopper On?"=w620:bool, "VISA Refnum out"=w621:refnum<visa-resource-name>)  [unwired: 6 in]
            n263 = local write "Chopper On"(w620) -> ()
            n264 = VISA Close(VISA resource name=w621, error in (no error)=w622) -> (error out=w619:errorcluster)
          }
          frame Enabled {
          }
        }
      }
    }
    n265 = case shown="True" "Auto Filter" {
      tunnel: [w229 w231] -> w213
      tunnel: w212 -> [w229 w230]
      frame False {
      }
      frame True {
        # "This is the timer for the filtering routine."
        n266 = call "Elapsed Time"("Time Target (s)"="Time Target (s)", "Auto Reset"=TRUE, "error in (no error)"=w230) -> ("Elapsed Time (s)"=w234:dbl, "Time has Elapsed"=w236:bool, "error out"=w235:errorcluster)  [unwired: 9 in, 5 out]
        "Time has Elapsed" <- w236
        n267 = Divide(x=w234, y=60.0) -> (x/y=→"Elapsed Time (min)":dbl)
        n268 = property on="Time has Elapsed" class="Bool (strict)"(error in=w235, "Val(Sgnl)"=w236) -> (error out=w231:errorcluster)  [unwired: 1 in, 1 out]
      }
    }
  }
  n269 = while {
    tunnel: w45 -> [w666]
    shift-right: [w663] -> _
    shift-left: w83 -> [w660]
    shift-right: [w662] -> _
    shift-left: w83 -> [w659]
    shift-right: [w661] -> _
    shift-left: w83 -> [w658]
    tunnel: w46 -> [w656]
    tunnel: "mic cal, scu" -> [w655]
    shift-right: [w653] -> w41
    shift-left: w33 -> [w652]
    shift-right: [w650] -> w40
    shift-left: w42 -> [w654]
    stop <- w657 stop-if-true
    # "Microphone Processing Loop (Consumer)"
    n270 = Dequeue Element(queue=w666) -> (element=w664:i32[][], error out=w665:errorcluster)  [unwired: 2 in, 2 out]
    n271 = case shown="No Error" w665 {
      selector: w665 -> [_ w697]
      tunnel: w664 -> [w690 _]
      tunnel: w660 -> [w694 w700]
      tunnel: w659 -> [w693 w698]
      tunnel: w658 -> [w692 w699]
      tunnel: [w670 w700] -> w663
      tunnel: [w669 w698] -> w662
      tunnel: [w668 w699] -> w661
      tunnel: [w667 w697] -> w657
      tunnel: w656 -> [w688 _]
      tunnel: w655 -> [w682 _]
      tunnel: [w671 T12 {"405 Mean"=0.0, "532 Mean"=0.0, "660 Mean"=0.0}] -> w651
      frame No Error {
        w695 = T13 0 items=["Rectangle"=0, "Hanning"=1, "Hamming"=2, "Blackman-Harris"=3, "Exact Blackman"=4, "Blackman"=5, "Flat Top"=6, "4 Term B-Harris "=7, "7 Term B-Harris"=8, "Low Sidelobe"=9, "Blackman Nuttall"=11, "Triangle"=30, "Bartlett-Hanning"=31, "Bohman"=32, "Parzen"=33, "Welch"=34, "Kaiser"=60, "Dolph-Chebyshev"=61, "Gaussian"=62] ("window")
        n272 = Index Array(array=w690, index (row)=0) -> (element=w689:i32[])  [unwired: 1 in]
        n273 = Bundle By Name("Y"=w689, "dt"=w688) -> (w687:waveform(i32))  [unwired: 1 in]
        "micwave" <- w687
        n274 = local read "320 F (Hz)"() -> (w685:i32)
        n275 = local read "375 F (Hz)"() -> (w684:i32)
        n276 = local read "445 F (Hz)"() -> (w683:i32)
        n277 = call-poly <vilib>:"FFT Spectrum (Mag-Phase).vi"("window"=w695, "time signal"=w687) -> ("error out"=w667:errorcluster, "magnitude"=w686:cluster{"f0":dbl, "df":dbl, "magnitude":dbl[]})  [unwired: 5 in, 3 out]
        "micfft" <- w686
        n278 = call-poly "fftGetMagsPoly.vi"("input cluster"=w686, "422 F (Hz)"=w685, "532 F (Hz)"=w684, "785 F (Hz)"=w683, "unit cal, scu"=w682) -> ("mag422 (mV)"=w677:dbl, "mag532 (mV)"=w676:dbl, "mag785 (mV)"=w675:dbl)  [unwired: 8 in]
        n279 = Bundle("X"=w694, "mag422 (mV)"=w677) -> (w681:cluster{"X":dbl[], "mag422 (mV) ":dbl})  [unwired: 1 in]
        n280 = Bundle("X"=w693, "mag532 (mV)"=w676) -> (w680:cluster{"X":dbl[], "mag532 (mV)":dbl})  [unwired: 1 in]
        n281 = Bundle("X"=w692, "mag785 (mV)"=w675) -> (w679:cluster{"X":dbl[], "mag785 (mV)":dbl})  [unwired: 1 in]
        n282 = call-poly "rollingAverage_multi.vi"("Magnitude Averaging (no. Avgs.)"="rollavg", "785nm"=w679, "532nm"=w680, "422nm"=w681) -> ("785nm Data"=w672:T14, "532nm Data"=w673:T15, "422nm Data"=w674:T16)  [unwired: 5 in]
        n283 = call-poly "micUnbundle.vi"("422nm Data"=w674, "532nm Data"=w673, "785nm Data"=w672) -> ("Output Cluster"=w671:T7, "422 New Array"=w670:dbl[], "532 New Array"=w669:dbl[], "785 New Array"=w668:dbl[])  [unwired: 9 in]
        "mic ts" <- w671
      }
      frame Error {
      }
    }
    n284 = Enqueue Element(queue=w652, element=w651, error in (no error)=w654) -> (queue out=w653:refnum<queue>, error out=w650:errorcluster)  [unwired: 1 in, 1 out]
  }
  n285 = while {
    shift-right: [w722] -> _
    shift-left: w83 -> [w719]
    shift-right: [w721] -> _
    shift-left: w83 -> [w718]
    shift-right: [w720] -> _
    shift-left: w83 -> [w717]
    tunnel: w49 -> [w715]
    tunnel: w46 -> [w714]
    tunnel: "mic cal, scu" -> [w713]
    shift-right: [w710] -> w38
    shift-left: w34 -> [w711]
    shift-right: [w709] -> w37
    shift-left: w39 -> [w712]
    shift-right: [w704] -> _
    shift-left: cluster{"f0":dbl, "df":dbl, "magnitude":dbl[]} {"f0"=0.0, "df"=0.0, "magnitude"=[]} ("magnitude") -> [w703]
    shift-right: [w701] -> _
    shift-left: "x" -> [w702]
    stop <- w716 stop-if-true
    # "Photodiode Processing Loop (Consumer)"
    n286 = Dequeue Element(queue=w715) -> (element=w723:i32[][], error out=w724:errorcluster)  [unwired: 2 in, 2 out]
    n287 = case shown="No Error" w724 {
      selector: w724 -> [_ w781]
      tunnel: w723 -> [w764 _]
      tunnel: w719 -> [w768 w784]
      tunnel: w718 -> [w767 w782]
      tunnel: w717 -> [w766 w783]
      tunnel: [w746 w784] -> w722
      tunnel: [w745 w782] -> w721
      tunnel: [w744 w783] -> w720
      tunnel: [w734 w781] -> w716
      tunnel: w714 -> [w762 _]
      tunnel: w713 -> [w757 _]
      tunnel: "660 PD Cal 3" -> [w741 _]
      tunnel: "532 PD Cal 3" -> [w742 _]
      tunnel: "405 PD Cal 3" -> [w743 _]
      tunnel: [w740 cluster{dbl, dbl, dbl} {0.0, 0.0, 0.0}] -> w708
      tunnel: [w728 w779] -> w704
      tunnel: w703 -> [w725 w779]
      tunnel: w702 -> [w736 w778]
      tunnel: [w726 w778] -> w701
      frame No Error {
        w769 = T13 0 items=["Rectangle"=0, "Hanning"=1, "Hamming"=2, "Blackman-Harris"=3, "Exact Blackman"=4, "Blackman"=5, "Flat Top"=6, "4 Term B-Harris "=7, "7 Term B-Harris"=8, "Low Sidelobe"=9, "Blackman Nuttall"=11, "Triangle"=30, "Bartlett-Hanning"=31, "Bohman"=32, "Parzen"=33, "Welch"=34, "Kaiser"=60, "Dolph-Chebyshev"=61, "Gaussian"=62] ("window")
        n288 = Unbundle(w725) -> ("f0"=w737:dbl, "df"=w738:dbl, "magnitude"=w733:dbl[])
        n289 = Index Array(array=w764, index (row)=0) -> (element=w763:i32[])  [unwired: 1 in]
        n290 = Bundle By Name("Y"=w763, "dt"=w762) -> (w761:waveform(i32))  [unwired: 1 in]
        "pdwave" <- w761
        n291 = local read "320 F (Hz)"() -> (w760:i32)
        n292 = local read "375 F (Hz)"() -> (w759:i32)
        n293 = local read "445 F (Hz)"() -> (w758:i32)
        n294 = call-poly <vilib>:"FFT Spectrum (Mag-Phase).vi"("window"=w769, "time signal"=w761) -> ("error out"=w735:errorcluster, "magnitude"=w739:cluster{"f0":dbl, "df":dbl, "magnitude":dbl[]})  [unwired: 5 in, 3 out]
        n295 = call-poly "fftGetMagsPoly.vi"("input cluster"=w725, "422 F (Hz)"=w760, "532 F (Hz)"=w759, "785 F (Hz)"=w758, "unit cal, scu"=w757) -> ("mag422 (mV)"=w752:dbl, "mag532 (mV)"=w751:dbl, "mag785 (mV)"=w750:dbl)  [unwired: 8 in]
        n296 = Increment(x=w736) -> (x+1=w727:dbl)
        n297 = Greater?(x=w727, y="y") -> (0:w729:bool)
        n298 = Bundle("X"=w768, "mag422 (mV)"=w752) -> (w756:cluster{"X":dbl[], "mag422 (mV) ":dbl})  [unwired: 1 in]
        n299 = Bundle("X"=w767, "mag532 (mV)"=w751) -> (w755:cluster{"X":dbl[], "mag532 (mV)":dbl})  [unwired: 1 in]
        n300 = Unbundle(w739) -> ("magnitude"=w731:dbl[])  [unwired: 2 out]
        n301 = Bundle("X"=w766, "mag785 (mV)"=w750) -> (w754:cluster{"X":dbl[], "mag785 (mV)":dbl})  [unwired: 1 in]
        n302 = case shown="False" w729 {
          tunnel: w735 -> [w774 w777]
          tunnel: [w774 w777] -> w734
          tunnel: w731 -> [w773 w776]
          tunnel: w733 -> [w772 _]
          tunnel: [w771 w776] -> w732
          tunnel: w727 -> [w770 _]
          tunnel: [w770 0.0 ("x")] -> w726
          frame False {
            n303 = Add(x=w772, y=w773) -> (x+y=w771:dbl[])
          }
          frame True {
          }
        }
        n304 = call-poly "rollingAverage_multi.vi"("Magnitude Averaging (no. Avgs.)"="Chart Rolling Average", "785nm"=w754, "532nm"=w755, "422nm"=w756) -> ("785nm Data"=w747:T14, "532nm Data"=w748:T15, "422nm Data"=w749:T16)  [unwired: 5 in]
        n305 = call-poly "pdNormalize.vi"("422 Data"=w749, "532 Data"=w748, "785 Data"=w747, "422 PD Cal 3"=w743, "532 PD Cal 3"=w742, "785 PD Cal 3"=w741) -> ("pd ts"=w740:cluster{dbl, dbl, dbl}, "422 New Array"=w746:dbl[], "532 New Array"=w745:dbl[], "785 New Array"=w744:dbl[])  [unwired: 5 in, 1 out]
        "pd ts" <- w740
        n306 = Bundle("f0"=w737, "df"=w738, "magnitude"=w732) -> (w728:cluster{"f0":dbl, "df":dbl, "magnitude":dbl[]})  [unwired: 1 in]
        "pdfft" <- w725
        "x 2" <- w736
      }
      frame Error {
      }
    }
    n307 = Enqueue Element(queue=w711, element=w708, error in (no error)=w712) -> (queue out=w710:refnum<queue>, error out=w709:errorcluster)  [unwired: 1 in, 1 out]
  }
  n308 = while {
    tunnel: w34 -> [w786]
    tunnel: w33 -> [w785]
    stop <- w792 stop-if-true
    # "Absorption Data Loop (Consummer II)"
    n309 = Dequeue Element(queue=w785) -> (element=w793:cluster{dbl, dbl, dbl}, error out=w791:errorcluster)  [unwired: 2 in, 2 out]
    n310 = Dequeue Element(queue=w786) -> (element=w788:cluster{dbl, dbl, dbl}, error out=w790:errorcluster)  [unwired: 2 in, 2 out]
    n311 = Wait (ms)(milliseconds to wait="save interval (ms)") -> ()  [unwired: 1 out]
    n312 = Merge Errors(w791, w790) -> (w789:errorcluster)
    n313 = case shown="No Error" w789 {
      selector: w789 -> [w830 w835]
      tunnel: w793 -> [w804 _]
      tunnel: [w817 w835] -> w792
      tunnel: w788 -> [w801 _]
      frame No Error {
        w794 = 0.0
        n314 = local read "tau0"() -> (w797:dbl)
        n315 = local read "tau"() -> (w795:dbl)
        n316 = Bundle("tau"=w795, "tau0"=w797) -> (w796:cluster{"tau":dbl, "tau0":dbl})  [unwired: 1 in]
        n317 = call-poly "absCalcPlot.vi"("CRD t, t0"=w796, "Cell Calibration, mV/mW"="cellcal", "Error In"=w830, "PD Values"=w801, "bkg values"="Bkg Values (mV)", "Mic Values"=w804) -> ("Error Out"=w818:errorcluster, "aae"=→"AAE":dbl, "Time Series"=→"abs/ext":cluster{dbl, dbl, dbl, "b_ext (1/Mm)":dbl}, "Spectrum"=→"Absorption Spectrum":cluster{dbl[], "Best Power Fit":dbl[]}[])  [unwired: 2 in]
        n318 = local read "Elapsed Time (min)"() -> (w807:dbl)
        n319 = local read "Filtering"() -> (w811:bool)
        n320 = local read "abs/ext"() -> (w816:cluster{dbl, dbl, dbl, "b_ext (1/Mm)":dbl})
        n321 = local read "mic ts"() -> (w822:T7)
        n322 = local read "pd ts"() -> (w829:cluster{dbl, dbl, dbl})
        n323 = local read "Calculated Resonance (Hz)"() -> (w812:dbl)
        n324 = Boolean To (0,1)(Boolean=w811) -> (0, 1=w810:i16)
        n325 = Unbundle(w822) -> ("422 Mean"=w821:dbl, "532 Mean"=w820:dbl, "785 Mean"=w819:dbl)
        n326 = Unbundle(w829) -> (w823:dbl, w824:dbl, w825:dbl)
        n327 = Unbundle(w816) -> (w815:dbl, w814:dbl, w813:dbl, "b_ext (1/Mm)"=w798:dbl)
        n328 = To Double Precision Float(number=w810) -> (double precision float=w809:dbl)
        n329 = Format Date/Time String(time format string (%c)="%Y-%m-%d %H:%M:%S\t") -> (date/time string=w826:string)  [unwired: 2 in]
        n330 = Format Into String(format string="%.4e\t%.4e\t%.4e\t%.4e\t%.4e\t%.4e\t%.4e\t%.4e\t%.4e\t%.4e\t%.4e\t%.4e\t%.4e\t%.4e\t%f\t%f\t%.1f", initial string=w826, error in=w818, w821, w820, w819, w794, w823, w824, w825, w794, w795, w815, w814, w813, w794, w798, w812, w809, w807) -> (resulting string=w808:string, error out=w817:errorcluster)
        n331 = local read "PAS Save"() -> (w805:bool)
        n332 = case shown="True" w805 {
          tunnel: w808 -> [_ w832]
          frame False {
          }
          frame True {
            n333 = local read "pas"() -> (w831:path)
            n334 = Build Array(w832) -> (w834:string[])
            n335 = call-poly <vilib>:"Write To Spreadsheet File.vi"("append to file? (new file:F)"=TRUE, "1D data"=w834, "file path (dialog if empty)"=w831) -> ()  [unwired: 5 in, 1 out]
          }
        }
      }
      frame Error {
      }
    }
  }
  n336 = call "PicoScope2000aClose.vi"("handle"=w30) -> ()  [unwired: 11 in]
  n337 = Release Queue(queue=w3, error in (no error)=w4) -> ()  [unwired: 1 in, 3 out]
  n338 = while {
    tunnel: w25 -> [w846]
    tunnel: w26 -> [w845]
    tunnel: w27 -> [w844]
    shift-right: [w843] -> _
    shift-left: _ -> [w842]
    tunnel: "factor" -> [w839]
    tunnel: w3 -> [w837]
    stop <- w840 stop-if-true
    # "CRD Processing Loop (Consumer)"
    n339 = Multiply(x=w846, y=w839) -> (x*y=w847:sgl)
    n340 = Dequeue Element(queue=w837, timeout in ms (-1)=1500) -> (element=w841:i16[][], error out=w838:errorcluster)  [unwired: 1 in, 2 out]
    n341 = case shown="No Error" w838 {
      selector: w838 -> [w853 w872]
      tunnel: w847 -> [w851 _]
      tunnel: w845 -> [w862 _]
      tunnel: w844 -> [w861 _]
      tunnel: [w860 w873] -> w843
      tunnel: w842 -> [w859 w873]
      tunnel: w841 -> [w858 _]
      tunnel: [w857 w872] -> w840
      frame No Error {
        w852 = 0
        n342 = call "picoCoAdd.vi"("error in (no error)"=w853, "Buffer In"=w858) -> ("error out"=w868:errorcluster, "Waveform Out"=w869:dbl[])  [unwired: 8 in]
        n343 = call "picoToVolts.vi"("error in (no error)"=w868, "Max_adc"=w862, "Range Index"=w861, "Data"=w869) -> ("error out"=w857:errorcluster, "Data (mV)"=w870:dbl[])  [unwired: 6 in]
        n344 = call "Get Tau.vi"("CalType"=analys_meth."DFT-5", "Dt"=w851, "X"=w870) -> ("B"=w854:dbl, "A"=w855:dbl, "tau"=w856:dbl)  [unwired: 5 in, 1 out]
        n345 = call "crdDisplayFit.vi"("N"=360, "B"=w854, "A"=w855, "tau"=w856) -> ("Fit Out"=w866:dbl[])  [unwired: 7 in]
        n346 = call "rollingAverage.vi"("No Avg"="tau Rolling Avg", "New Element"=w856, "Rolling Array"=w859) -> ("mean"=→"tau":dbl, "New Array"=w860:dbl[])  [unwired: 6 in, 1 out]
        n347 = Bundle(w852, w851, "Data (mV)"=w870) -> (w871:cluster{i32, sgl, "Data (mV)":dbl[]})  [unwired: 1 in]
        n348 = Bundle(w852, 1e-06, "Fit Out"=w866) -> (w864:cluster{i32, dbl, "Fit Out":dbl[]})  [unwired: 1 in]
        n349 = Build Array(w864, w871) -> (→"decay":cluster{i32, dbl, "Data (mV)":dbl[]}[])
      }
      frame Error {
      }
    }
  }
  n350 = Release Queue(queue=w41, error in (no error)=w40) -> ()  [unwired: 1 in, 3 out]
  n351 = Merge Errors(w91, w81) -> (w90:errorcluster)
  n352 = Release Queue(queue=w38, error in (no error)=w37) -> ()  [unwired: 1 in, 3 out]
  n353 = call <vilib>:"Simple Error Handler.vi"("error in (no error)"=w90) -> ("error out"=w89:errorcluster)  [unwired: 4 in, 4 out]
  n354 = flat-sequence {
    tunnel: w89 -> [w874]
    tunnel: [w874] -> w88
    frame #0 {
      n355 = local write "Exit"(FALSE) -> ()
    }
  }
  "Error Console" <- w88
